vi "TI sbRIO Main (FPGA) (CMFB first try).vi"() -> ()   [LabVIEW 2019]
uses:
  <userlib>/_NI SPI IP/FPGA/Controllers/Public/Transfer Settings.ctl
  Type Defs/Diagnostic Mode.ctl
  Controls/SPI Channels.ctl
  <vilib>/Platform/TimedLoop/XDataNode/timing_clust.ctl
  <vilib>/Platform/TimedLoop/XDataNode/nitl_modes.ctl
  <vilib>/Platform/TimedLoop/XDataNode/wakeup.ctl
  <vilib>/rvi/FXPMathLib/FxpDiv/subVIs/nifxpmath_Div_SimConfig.ctl
  <vilib>/rvi/FXPMathLib/basic elements/FxpIntAccumulator/subVIs/nifxpmath_IntAccumulator_SimConfig.ctl
  <vilib>/rvi/FXPMathLib/FxpSqrt/subVIs/nifxpmath_Sqrt_SimConfig.ctl
  <vilib>/fxp/LVFixedPointOverflowPolicyTypeDef.ctl
  <userlib>/_NI SPI IP/FPGA/Controllers/Public/Spi Master Inputs.ctl
  <vilib>/rvi/Emulation/niFpgaGetClockAttributes.vi
  <vilib>/rvi/Emulation/niFpgaSctlEmulationGetInTimedLoop.vi
  <vilib>/rvi/Emulation/niFpgaEmulationReportErrorSimple.vi
  <vilib>/rvi/eio/common/nirviEmuTemplateMethod_errors.vi
  Onboard AIs Global.vi
  <vilib>/rvi/Emulation/niFpgaProcessEmulError.vi
  <vilib>/rvi/Emulation/niFpgaCriticalErrorInLSC.vi
  ADC AI Global.vi
  <vilib>/rvi/FXPMathLib/FxpDiv/simVIs/DllFxpDivTemp_sub.vi
  <vilib>/rvi/DataTransferAndStorage/Container/Common/niFpgaContainerExecOnDevCompGetState.vi
  <vilib>/rvi/Emulation/niFpgaEmulationIsFPGAContextNoSignature.vi
  <vilib>/rvi/errors/niFpgaSetErrorForExecOnDevCompSimple.vi
  <vilib>/rvi/eio/common/nirviEmuReportErrorAndStop.vi
  <vilib>/rvi/DataTransferAndStorage/Container/Common/niFpgaContainerGetUniqueNameForEmu.vi
  <vilib>/rvi/FIFO/Fifo_Resource/nirvififoEmulationSetSize.vi
  <vilib>/rvi/FIFO/Fifo_Resource/nirviFifoEmulationQueueMgr.vi
  <instcachedir>/0/nirviFifoEmulationQueueMgr_E5CAEC123FF24DC58D834DCA3CDAA9B5.lvgen/nirviFifoEmulationQueueMgr_E5CAEC123FF24DC58D834DCA3CDAA9B5_000.vi
  <vilib>/rvi/FIFO/Fifo_Resource/nirvififoEmulationDetermineInputValidOut.vi
  <vilib>/rvi/FIFO/Fifo_Resource/nirvififoEmulationCreateLock.vi
  <vilib>/rvi/FIFO/Fifo_Resource/nirvififoEmulationObtainLock.vi
  <vilib>/rvi/FIFO/Fifo_Resource/nirvififoEmulationReleaseLock.vi
  <vilib>/rvi/occurrence/nirviWaitOnOccurrenceBase.vi
  <vilib>/rvi/errors/nirviReportUnexpectedCaseInternalError.vi
  <vilib>/rvi/errors/nirviReportUnexpectedCaseInternalError (U32).vi
  <vilib>/Utility/error.llb/Clear Errors.vi
  <vilib>/rvi/interface/RandomDataEmulation/niFpgaRandomDataHandleErrors.vi
  Flow Frequencies Global.vi
  ADC AI Global (Avg).vi
  <vilib>/rvi/Analysis/common/codeGenErrors/XNode/niFpgaXNodeCodeGenErrorHandle.vi
  <vilib>/rvi/FXPMathLib/basic elements/FxpIntAccumulator/simVIs/DllFxpIntAccumulator_sub.vi
  <vilib>/rvi/FXPMathLib/FxpSqrt/simVIs/DllSqrtTemp_sub.vi
  Pump Currents Global.vi
  Diagnostic Global.vi
  <vilib>/eio/EIONode/EIONode.xnode
  <vilib>/rvi/FXPMathLib/FxpDiv/XNode/nifxpmath_Div.xnode
  <vilib>/rvi/DataTransferAndStorage/Container/XNode/niFpgaContainer.xnode
  <vilib>/rvi/FIFO/Fifo_Resource/niFpgaFifoEmulationRefIn.vi
  <vilib>/rvi/FXPMathLib/FxpMul/XNode/nifxpmath_Multiplier.xnode
  <vilib>/rvi/FXPMathLib/FxpAdd/XNode/nifxpmath_Add.xnode
  <vilib>/rvi/Analysis/measure/butterworth/XNode/niFpgaButterworthFilter.xnode
  <vilib>/rvi/Analysis/measure/dc-rms/XNode/niFpgaDC-RMS.xnode
  <vilib>/Platform/TimedLoop/XDataNode/XDataNode.xnode
  <vilib>/rvi/FXPMathLib/basic elements/FxpIntAccumulator/XNode/nifxpmath_IntAccumulator.xnode
  <vilib>/rvi/FXPMathLib/FxpSqrt/XNode/nifxpmath_Sqrt.xnode
  <vilib>/rvi/interface/RandomDataEmulation/nirviRandomDataFpgaReadWriteTemplate.vi
  <vilib>/eio/EIOMethodNode/EIOMethodNode.xnode
  <vilib>/rvi/FXPMathLib/sim/FxpSim.dll
  <vilib>/Platform/TimedLoop/XDataNode/XDNodeRunTimeDep.lvlib
  <userlib>/_NI SPI IP/FPGA/Controllers/NI SPI IP FPGA.lvlib
panel:
  out "Restarts":i32[](array[numeric])
  out "Cmd Pump Starts":u32[](array[numeric])
  in  "Stop Command":i32
  in  "Initial Cmd Starts":u32[](array[numeric])=[0, 0, 0, 0, 0, 0]
  in  "Ctrl Currents":fxp<+/-,28,17>[](array[numeric])=[0.0, 0.0, 0.0, 0.0, 0.0, 0.0]
  in  "Initial Acutal Starts":u32[](array[numeric])=[0, 0, 0, 0, 0, 0]
  in  "Power Relays":bool[](array[boolean])=[FALSE, FALSE, FALSE, FALSE, FALSE, FALSE]
  out "Actual Pump Starts":u32[](array[numeric])
  out "Timers (ms)":u32[](array[numeric])
  out "Pump On States":bool[](array[boolean])
  in  "Off Current Thresh":fxp<+/-,28,17>
  in  "Min Off Time":u32
  in  "On Current Thresh":fxp<+/-,28,17>
  in  "Min On Time":u32
  in  "Reset Pump Starts":bool
  in  "Pump Starts Enable":bool
  in  "Diag Max Period (ticks)":u32
  in  "Diagnostic Mode":T1=enum."PSA"
  in  "Duty (Ticks)":i32[](array[numeric])=[0, 0, 0, 0, 0, 0]
  out "Elapsed Times OUT":fxp<+,40,40>[](array[numeric])
  out "Data OUT":fxp<+/-,28,17>[](array[numeric])
  in  "Diagnostic Filter":u16=5
  in  "Invert Diagnostic":bool
  in  "Diagnostic Freq Coeff":i32
  in  "Count Off-Time":bool
  in  "Elapsed Times":fxp<+,40,40>[](array[numeric])=[0.0, 0.0, 0.0, 0.0, 0.0, 0.0]
  in  "ADC Init":bool=TRUE
  in  "FFT_Amp?":bool=TRUE
  in  "Max Period (ticks)":u32
  in  "Freq Flow?":bool
  in  "Divide Value":u8=1
  in  "Current Threshold":fxp<+,26,7>=1.0 format="%#_22g"
  in  "Enable Timers":bool[](array[boolean])=[FALSE, FALSE, FALSE, FALSE, FALSE, FALSE]
  in  "PumpCurrentM":fxp<+/-,16,9>=-60.0 format="%#_25g"
  in  "PumpCurrentB":fxp<+/-,16,9>=-60.0 format="%#_25g"
  in  "InvertPWM?":bool
  in  "DIO25":bool
  in  "DIO24":bool
  out "DIO23":bool
  in  "DIO22":bool
  in  "DIO21":bool
  in  "DIO20":bool
  in  "DIO19":bool
  in  "DIO18":bool
  in  "DIO17":bool
  in  "DIO16":bool
  in  "DIO15":bool
  in  "DIO14":bool
  in  "DIO13":bool
  in  "DIO12":bool
  out "ADC Read Data":u64 format="%.0x"
  in  "ADC CS Mode":enum16{"All", "CS0", "CS1"}(ring)
  in  "ADC Trigger":bool=TRUE
  in  "ADC SPI Settings":T2 {"Direction Change Bit" max=64 step=1; "Transfer Length (bits)" min=1 max=64 step=1}
  in  "ADC Data In":u64 format="%.0x"
  in  "ADC Conversion Request":bool
  in  "ADC Manual":bool
  in  "Brushless":bool
  in  "AI Divisor":u32
  in  "AO3":fxp<+/-,20,5>
  in  "AO2":fxp<+/-,20,5>
  in  "Pressure Cmd":fxp<+/-,20,5>
  in  "PS Cmd":fxp<+/-,20,5>
  in  "Loop Timer (uSec)":u32=100
  in  "Timer Resets":bool[](array[boolean])=[FALSE, FALSE, FALSE, FALSE, FALSE, FALSE]
  in  "PWM Period (Ticks)":u32=40000000
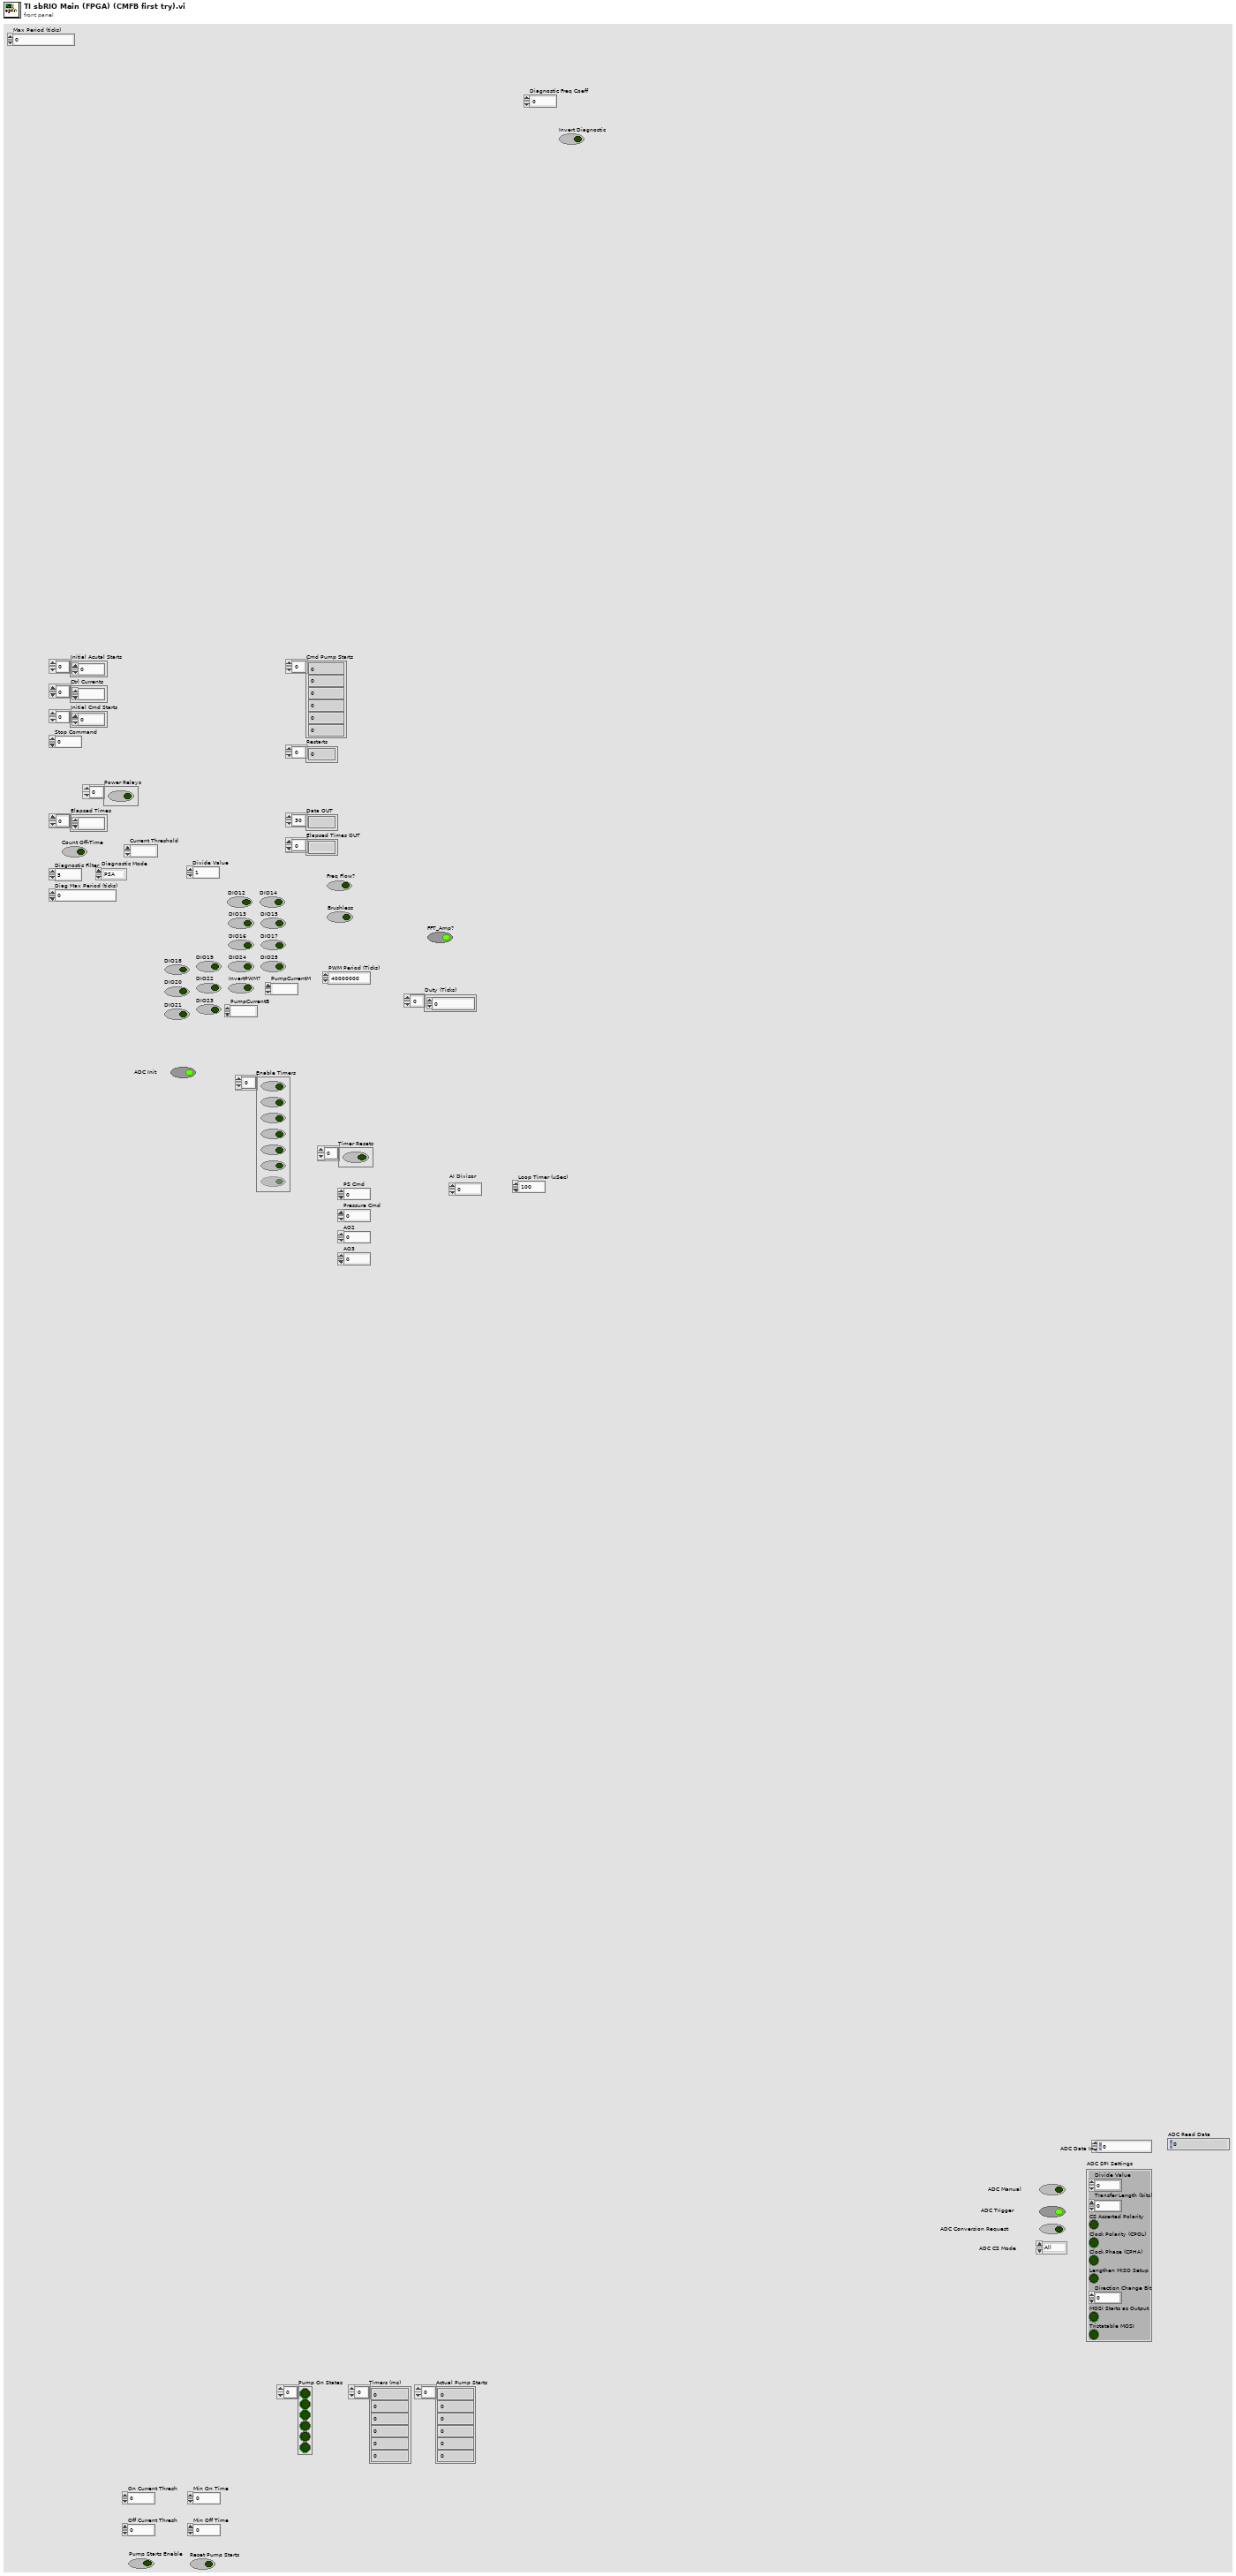
[diagram p1: front panel]
types:
  T1 = typedef "Diagnostic Mode.ctl" = enum16{"None", "PSA", "CMFB"}
  T2 = typedef "NI SPI IP FPGA.lvlib/Transfer Settings.ctl" = cluster{"Divide Value":u8, "Transfer Length (bits)":u8, "CS Asserted Polarity":bool, "Clock Polarity (CPOL)":bool, "Clock Phase (CPHA)":bool, "Lengthen MISO Setup":bool, "Direction Change Bit":u8, "MOSI Starts as Output":bool, "Tristatable MOSI":bool}
  T3 = typedef "SPI Channels.ctl" = cluster{"CS":refnum<k21>, "CLK":refnum<k21>, "MOSI":refnum<k21>, "MISO":refnum<k21>}
  T4 = typedef "XDNodeRunTimeDep.lvlib/timing_clust.ctl" = cluster{"Expected End [f-1]":u64, "Actual End [f-1]":u64, "Finished Late? [f-1]":bool, "Expected End [i-1]":u64, "Actual End [i-1]":u64, "Finished Late? [i-1]":bool, "Expected Start [i]":u64, "Actual Start [i]":u64, "Expected Start [f]":u64, "Actual Start [f]":u64, "Source Name":string, "Structure Name":string, "Period":i64, "Deadline":i64, "Offset":i64, "Start":i64, "Priority":i32, "Timeout":i32, "Mode":T5, "Wakeup Reason":T6, "Error":errorcluster, "Source Type":string, "Secondary Source Type":string, "Global End Time":u64, "Global Start Time":u64, "Frame Duration":u64, "Iteration Duration":u64, "Assigned CPU":i32, "I/O Scan Engine Mode":u32}
  T5 = typedef "XDNodeRunTimeDep.lvlib/nitl_modes.ctl" = enum32{"No Change", "Process missed periods, maintain original phase", "Discard missed periods, maintain original phase", "Process missed periods, ignore original phase", "Discard missed periods, ignore original phase"}
  T6 = typedef "XDNodeRunTimeDep.lvlib/wakeup.ctl" = enum32{"Normal", "Aborted", "Asynchronous wakeup", "Timing source error", "Timed loop error", "Timeout"}
  T7 = typedef "NI SPI IP FPGA.lvlib/Spi Master Inputs.ctl" = cluster{"MISO":bool}
  T8 = typedef "NI SPI IP FPGA.lvlib/Spi Master Outputs.ctl" = cluster{"Chip Select":bool, "Clock":bool, "MOSI":bool, "MOSI OE":bool}
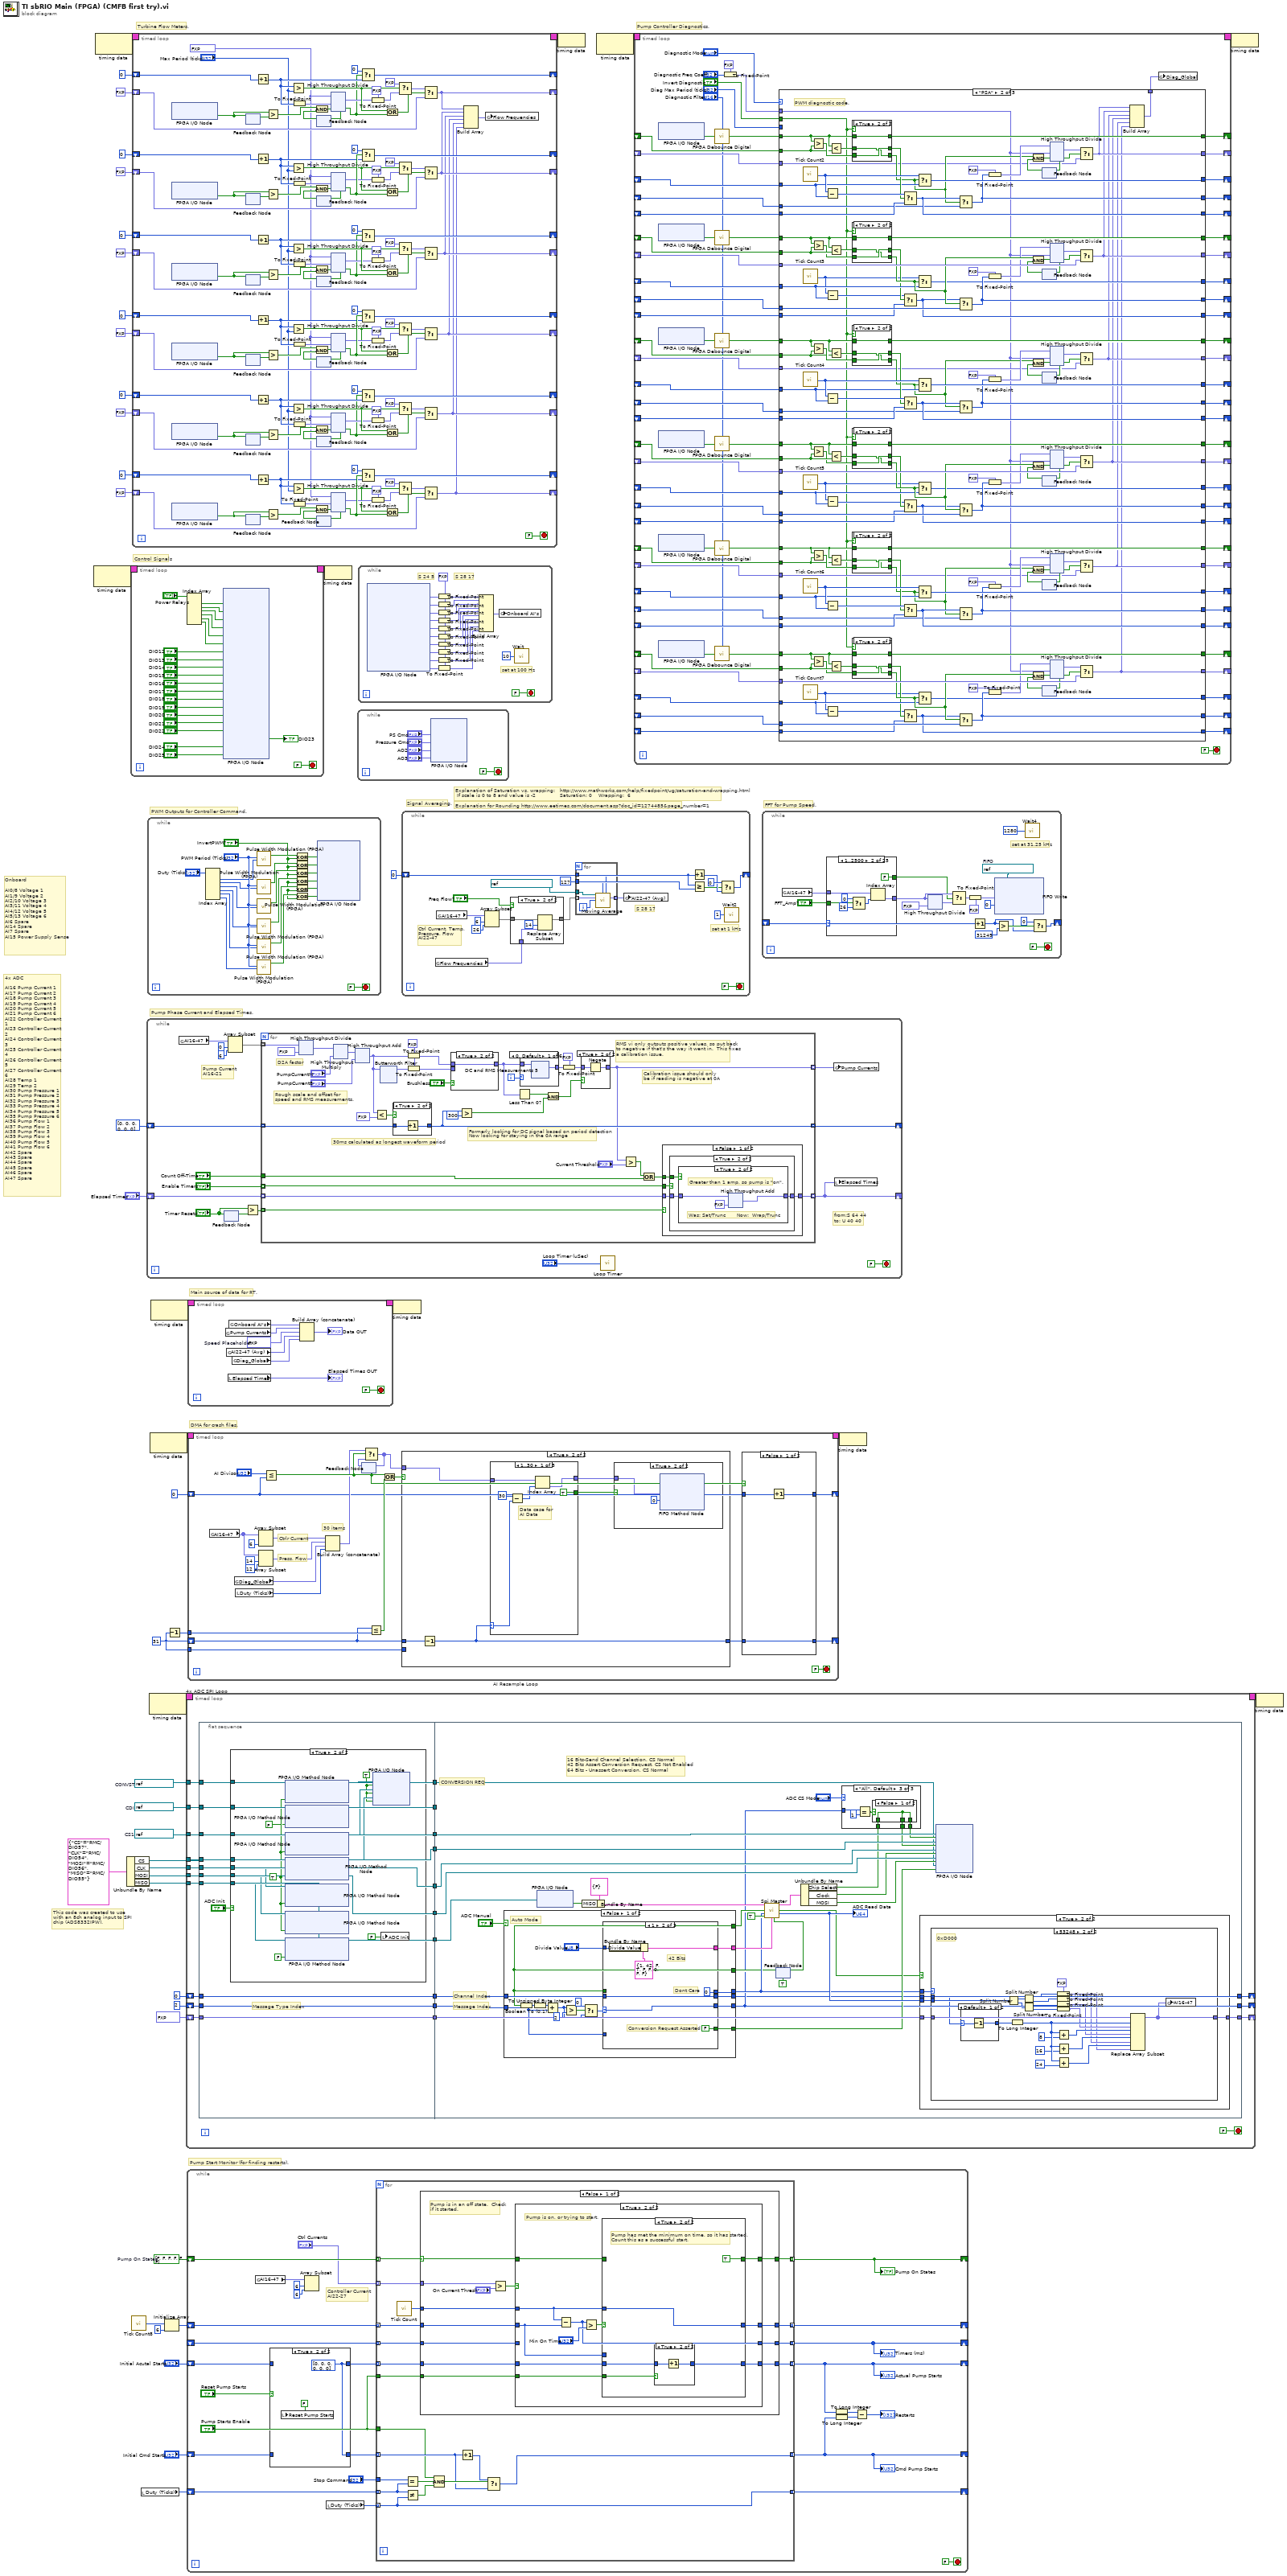
[diagram p0: block diagram]
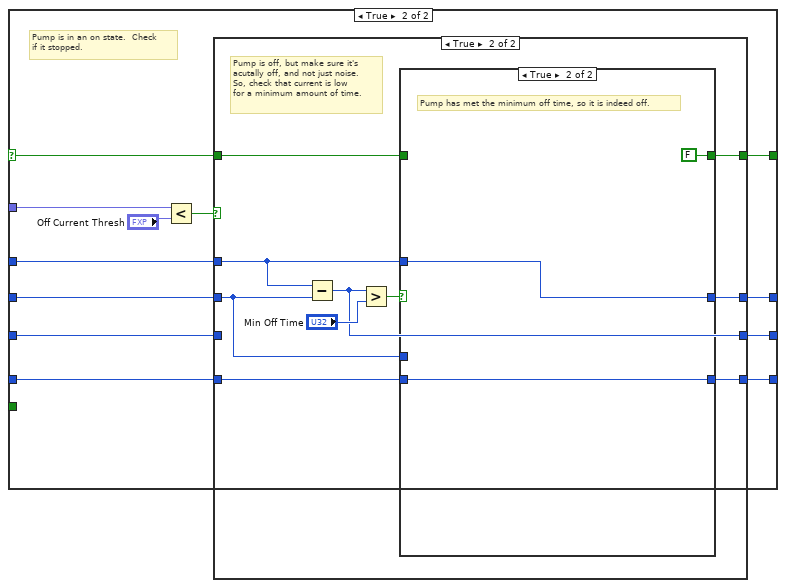
[diagram p6: hidden frame]
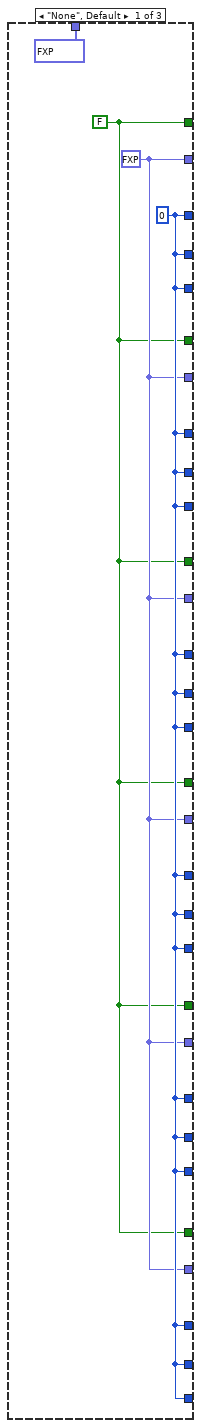
[diagram p9: hidden frame]
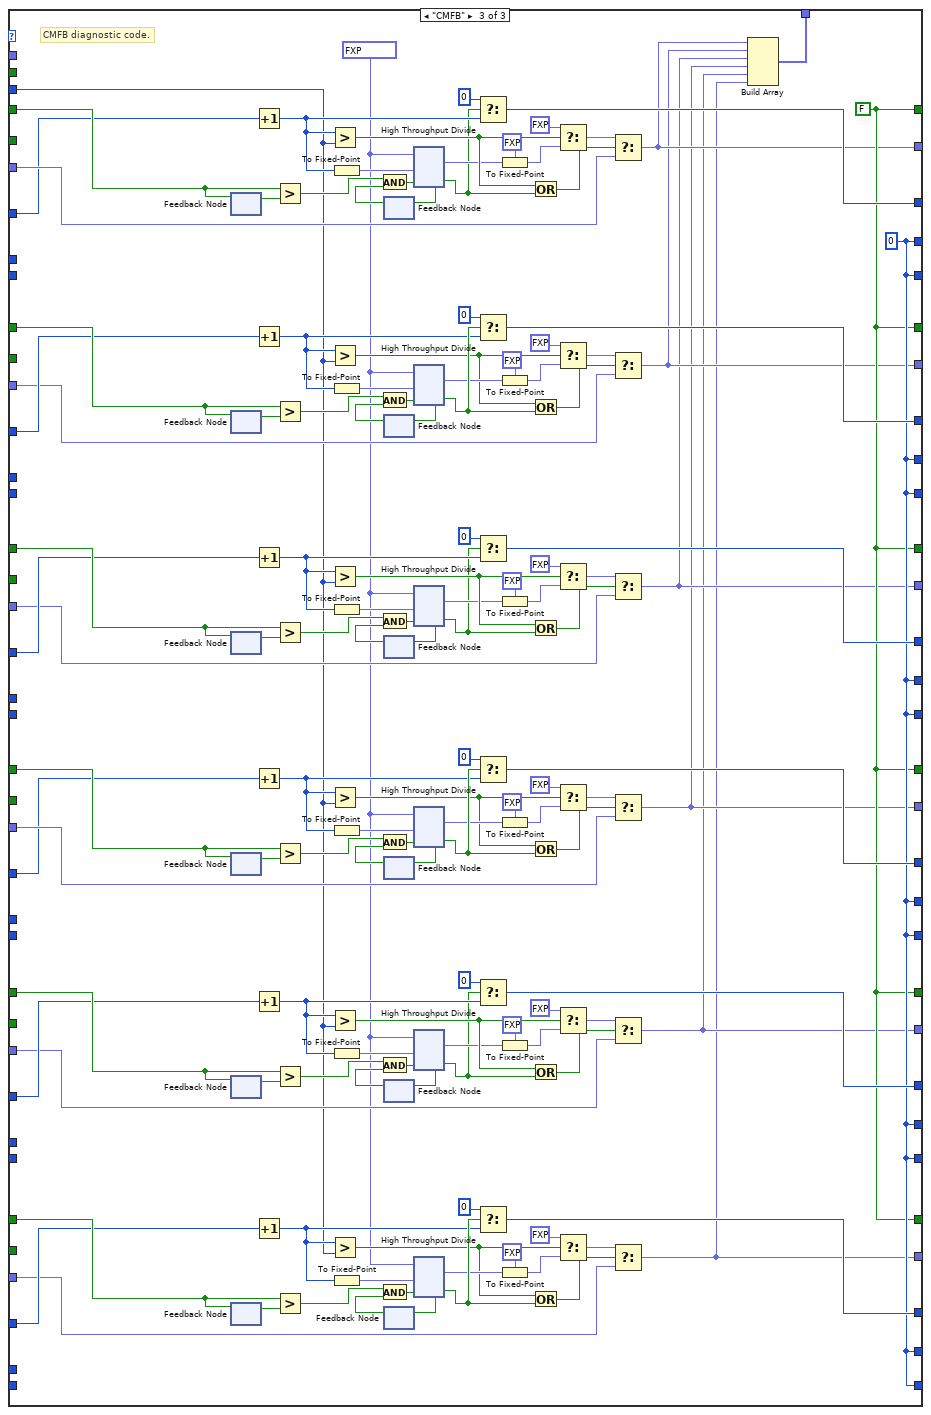
[diagram p16: hidden frame]
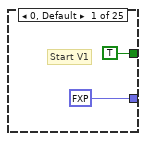
[diagram p17: hidden frame]
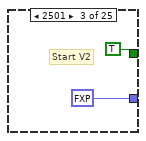
[diagram p18: hidden frame]
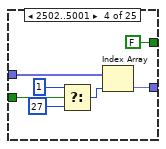
[diagram p19: hidden frame]
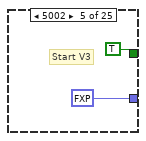
[diagram p20: hidden frame]
diagram:
  w7 = bool[] [FALSE, FALSE, FALSE, FALSE, FALSE, FALSE]  # Pump On States
  w38 = refnum<k21> "RMC/DIO60"  # CONVST
  w39 = refnum<k21> "RMC/DIO59"  # CDI
  w40 = refnum<k21> "RMC/DIO58"  # CS1
  w44 = u8 31 ("Sample Divisor")
  # "Pump Start Monitor (for finding restarts)."
  # "DMA for crash files."
  # "Main source of data for RT."
  # "Pump Phase Current and Elapsed Times."
  # "PWM Outputs for Controller Command."
  # "Signal Averaging."
  # "FFT for Pump Speed."
  # "Pump Controller Diagnostics."
  # "Turbine Flow Meters."
  # "Control Signals"
  # "4x ADC\n\nAI16\tPump Current 1\nAI17\tPump Current 2\nAI18\tPump Current 3\nAI19\tPump Current 4\nAI20\tPump Current 5\nAI21\tPump Current 6\nAI22\tController Current 1\nAI23\tController Current 2\nAI24\tController Current 3\nAI25\tController Current 4\nAI26\tController Current 5\nAI27\tController Current 6\nAI28\tTemp 1\nAI29\tTemp 2\nAI30\tPump Pressure 1\nAI31\tPump Pressure 2\nAI32\tPump Pressure 3\nAI33\tPump Pressure 4\nAI34\tPump Pressure 5\nAI35\tPump Pressure 6\nAI36\tPump Flow 1\nAI37\tPump Flow 2\nAI38\tPump Flow 3\nAI39\tPump Flow 4\nAI40\tPump Flow 5\nAI41\tPump Flow 6\nAI42\tSpare\nAI43\tSpare\nAI44\tSpare\nAI45\tSpare\nAI46\tSpare\nAI47\tSpare"
  # "Onboard\n\nAI0/8\tVoltage 1\nAI1/9\tVoltage 2\nAI2/10\tVoltage 3\nAI3/11\tVoltage 4\nAI4/12\tVoltage 5\nAI5/13\tVoltage 6\nAI6\tSpare\nAI14\tSpare\nAI7\tSpare\nAI15\tPower Supply Sense"
  # "This code was created to use\nwith an 8ch analog input to SPI\nchip (ADS8332IPW)."
  # "Explanation for Rounding http://www.eetimes.com/document.asp?doc_id=1274485&page_number=1"
  # "Explanation of Saturation vs. wrapping:   http://www.mathworks.com/help/fixedpoint/ug/saturation-and-wrapping.html\n If scale is 0 to 8 and value is -2               Saturation: 0    Wrapping:  6"
  n1 = node-c288() -> (w29:T4)  [unwired: 1 in]
  n2 = node-c288() -> (w27:T4)  [unwired: 1 in]
  n3 = Unbundle By Name(T3 {"CS"="RMC/DIO57", "CLK"="RMC/DIO54", "MOSI"="RMC/DIO56", "MISO"="RMC/DIO55"} ("SPI Channels")) -> ("CS"=w31:refnum<k21>, "CLK"=w32:refnum<k21>, "MOSI"=w33:refnum<k21>, "MISO"=w34:refnum<k21>)
  n4 = timed-loop {
    timing: w29 -> [_]
    timing-out: [_] -> w28
    stop <- FALSE stop-if-true
    n5 = Index Array(array="Power Relays") -> (element #1=w54:bool, element #2=w53:bool, element #3=w52:bool, element #4=w51:bool, element #5=w50:bool, element #6=w49:bool)  [unwired: 6 in]
    n6 = xnode "FPGA I/O Node"("RMC/DIO6"=w54, "RMC/DIO7"=w53, "RMC/DIO8"=w52, "RMC/DIO9"=w51, "RMC/DIO10"=w50, "RMC/DIO11"=w49, "RMC/DIO12"="DIO12", "RMC/DIO13"="DIO13", "RMC/DIO14"="DIO14", "RMC/DIO15"="DIO15", "RMC/DIO16"="DIO16", "RMC/DIO17"="DIO17", "RMC/DIO18"="DIO18", "RMC/DIO19"="DIO19", "RMC/DIO20"="DIO20", "RMC/DIO21"="DIO21", "RMC/DIO22"="DIO22", "RMC/DIO24"="DIO24", "RMC/DIO25"="DIO25") -> ("RMC/DIO23"=→"DIO23":bool)  [unwired: 21 in, 21 out]
  }
  n7 = call "Tick Count8"() -> ("Tick Count(mSec)"=w3:u32)
  n8 = timed-loop {
    timing: w27 -> [_]
    timing-out: [_] -> w26
    shift-right: [w197] -> _
    shift-left: u32 0 ("f") -> [w196]
    shift-right: [w79] -> _
    shift-left: fxp<+/-,28,17> 0.0 ("AI0") -> [w191]
    shift-right: [w166] -> _
    shift-left: u32 0 ("f") -> [w167]
    shift-right: [w78] -> _
    shift-left: fxp<+/-,28,17> 0.0 ("AI0") -> [w172]
    shift-right: [w157] -> _
    shift-left: u32 0 ("f") -> [w156]
    shift-right: [w77] -> _
    shift-left: fxp<+/-,28,17> 0.0 ("AI0") -> [w151]
    shift-right: [w126] -> _
    shift-left: u32 0 ("f") -> [w127]
    shift-right: [w76] -> _
    shift-left: fxp<+/-,28,17> 0.0 ("AI0") -> [w132]
    shift-right: [w117] -> _
    shift-left: u32 0 ("f") -> [w116]
    shift-right: [w75] -> _
    shift-left: fxp<+/-,28,17> 0.0 ("AI0") -> [w111]
    shift-right: [w86] -> _
    shift-left: u32 0 ("f") -> [w87]
    shift-right: [w74] -> _
    shift-left: fxp<+/-,28,17> 0.0 ("AI0") -> [w92]
    stop <- FALSE stop-if-true
    w81 = fxp<+,32,32> 40000000.0 ("x")
    n9 = xnode "FPGA I/O Node"() -> ("RMC/DIO32"=w201:bool)  [unwired: 1 in, 1 out]
    n10 = xnode "FPGA I/O Node"() -> ("RMC/DIO33"=w162:bool)  [unwired: 1 in, 1 out]
    n11 = xnode "FPGA I/O Node"() -> ("RMC/DIO34"=w161:bool)  [unwired: 1 in, 1 out]
    n12 = xnode "FPGA I/O Node"() -> ("RMC/DIO35"=w122:bool)  [unwired: 1 in, 1 out]
    n13 = xnode "FPGA I/O Node"() -> ("RMC/DIO36"=w121:bool)  [unwired: 1 in, 1 out]
    n14 = xnode "FPGA I/O Node"() -> ("RMC/DIO37"=w82:bool)  [unwired: 1 in, 1 out]
    n15 = feedback-in #1(w201) -> ()
    n16 = feedback #1() -> (w200:bool)  [unwired: 1 in]
    n17 = feedback #2() -> (w163:bool)  [unwired: 1 in]
    n18 = feedback-in #2(w162) -> ()
    n19 = feedback #3() -> (w160:bool)  [unwired: 1 in]
    n20 = feedback-in #3(w161) -> ()
    n21 = feedback #4() -> (w123:bool)  [unwired: 1 in]
    n22 = feedback-in #4(w122) -> ()
    n23 = feedback #5() -> (w120:bool)  [unwired: 1 in]
    n24 = feedback-in #5(w121) -> ()
    n25 = feedback #6() -> (w83:bool)  [unwired: 1 in]
    n26 = feedback-in #6(w82) -> ()
    n27 = Increment(x=w196) -> (x+1=w195:u32)
    n28 = Increment(x=w167) -> (x+1=w168:u32)
    n29 = Increment(x=w156) -> (x+1=w155:u32)
    n30 = Increment(x=w127) -> (x+1=w128:u32)
    n31 = Increment(x=w116) -> (x+1=w115:u32)
    n32 = Increment(x=w87) -> (x+1=w88:u32)
    n33 = Greater?(x=w201, y=w200) -> (0:w182:bool)
    n34 = Greater?(x=w162, y=w163) -> (0:w181:bool)
    n35 = Greater?(x=w161, y=w160) -> (0:w142:bool)
    n36 = Greater?(x=w122, y=w123) -> (0:w141:bool)
    n37 = Greater?(x=w121, y=w120) -> (0:w102:bool)
    n38 = Greater?(x=w82, y=w83) -> (0:w101:bool)
    n39 = Greater?(x=w195, y="Max Period (ticks)") -> (0:w199:bool)
    n40 = Greater?(x=w168, y="Max Period (ticks)") -> (0:w164:bool)
    n41 = Greater?(x=w155, y="Max Period (ticks)") -> (0:w159:bool)
    n42 = Greater?(x=w128, y="Max Period (ticks)") -> (0:w124:bool)
    n43 = Greater?(x=w115, y="Max Period (ticks)") -> (0:w119:bool)
    n44 = Greater?(x=w88, y="Max Period (ticks)") -> (0:w84:bool)
    n45 = To Fixed-Point(number=w195) -> (fixed-point=w194:fxp<+,32,32>)  [unwired: 1 in]
    n46 = To Fixed-Point(number=w168) -> (fixed-point=w169:fxp<+,32,32>)  [unwired: 1 in]
    n47 = To Fixed-Point(number=w155) -> (fixed-point=w154:fxp<+,32,32>)  [unwired: 1 in]
    n48 = To Fixed-Point(number=w128) -> (fixed-point=w129:fxp<+,32,32>)  [unwired: 1 in]
    n49 = To Fixed-Point(number=w115) -> (fixed-point=w114:fxp<+,32,32>)  [unwired: 1 in]
    n50 = To Fixed-Point(number=w88) -> (fixed-point=w89:fxp<+,32,32>)  [unwired: 1 in]
    n51 = feedback #7() -> (w183:bool)  [unwired: 1 in]
    n52 = And(x=w182, y=w183) -> (x .and. y?=w184:bool)
    n53 = feedback #8() -> (w180:bool)  [unwired: 1 in]
    n54 = And(x=w181, y=w180) -> (x .and. y?=w179:bool)
    n55 = feedback #9() -> (w143:bool)  [unwired: 1 in]
    n56 = And(x=w142, y=w143) -> (x .and. y?=w144:bool)
    n57 = feedback #10() -> (w140:bool)  [unwired: 1 in]
    n58 = And(x=w141, y=w140) -> (x .and. y?=w139:bool)
    n59 = feedback #11() -> (w103:bool)  [unwired: 1 in]
    n60 = And(x=w102, y=w103) -> (x .and. y?=w104:bool)
    n61 = feedback #12() -> (w100:bool)  [unwired: 1 in]
    n62 = And(x=w101, y=w100) -> (x .and. y?=w99:bool)
    n63 = xnode "High Throughput Divide"("x"=w81, "y"=w194, "input valid"=w184) -> ("x/y"=w190:fxp<+,28,17>, "output valid"=w186:bool, "ready for input"=w185:bool)  [unwired: 1 in]
    n64 = feedback-in #7(w185) -> ()
    n65 = xnode "High Throughput Divide"("x"=w81, "y"=w169, "input valid"=w179) -> ("x/y"=w173:fxp<+,28,17>, "output valid"=w177:bool, "ready for input"=w178:bool)  [unwired: 1 in]
    n66 = feedback-in #8(w178) -> ()
    n67 = xnode "High Throughput Divide"("x"=w81, "y"=w154, "input valid"=w144) -> ("x/y"=w150:fxp<+,28,17>, "output valid"=w146:bool, "ready for input"=w145:bool)  [unwired: 1 in]
    n68 = feedback-in #9(w145) -> ()
    n69 = xnode "High Throughput Divide"("x"=w81, "y"=w129, "input valid"=w139) -> ("x/y"=w133:fxp<+,28,17>, "output valid"=w137:bool, "ready for input"=w138:bool)  [unwired: 1 in]
    n70 = feedback-in #10(w138) -> ()
    n71 = xnode "High Throughput Divide"("x"=w81, "y"=w114, "input valid"=w104) -> ("x/y"=w110:fxp<+,28,17>, "output valid"=w106:bool, "ready for input"=w105:bool)  [unwired: 1 in]
    n72 = feedback-in #11(w105) -> ()
    n73 = xnode "High Throughput Divide"("x"=w81, "y"=w89, "input valid"=w99) -> ("x/y"=w93:fxp<+,28,17>, "output valid"=w97:bool, "ready for input"=w98:bool)  [unwired: 1 in]
    n74 = feedback-in #12(w98) -> ()
    n75 = Select(t=u32 0 ("f"), s=w186, f=w195) -> (s? t:f=w197:u32)
    n76 = Select(t=u32 0 ("f"), s=w177, f=w168) -> (s? t:f=w166:u32)
    n77 = Select(t=u32 0 ("f"), s=w146, f=w155) -> (s? t:f=w157:u32)
    n78 = Select(t=u32 0 ("f"), s=w137, f=w128) -> (s? t:f=w126:u32)
    n79 = Select(t=u32 0 ("f"), s=w106, f=w115) -> (s? t:f=w117:u32)
    n80 = Select(t=u32 0 ("f"), s=w97, f=w88) -> (s? t:f=w86:u32)
    n81 = To Fixed-Point(fixed-point type=fxp<+/-,28,17> 0.0 ("AI0"), number=w190) -> (fixed-point=w188:fxp<+/-,28,17>)
    n82 = To Fixed-Point(fixed-point type=fxp<+/-,28,17> 0.0 ("AI0"), number=w173) -> (fixed-point=w175:fxp<+/-,28,17>)
    n83 = To Fixed-Point(fixed-point type=fxp<+/-,28,17> 0.0 ("AI0"), number=w150) -> (fixed-point=w148:fxp<+/-,28,17>)
    n84 = To Fixed-Point(fixed-point type=fxp<+/-,28,17> 0.0 ("AI0"), number=w133) -> (fixed-point=w135:fxp<+/-,28,17>)
    n85 = To Fixed-Point(fixed-point type=fxp<+/-,28,17> 0.0 ("AI0"), number=w110) -> (fixed-point=w108:fxp<+/-,28,17>)
    n86 = To Fixed-Point(fixed-point type=fxp<+/-,28,17> 0.0 ("AI0"), number=w93) -> (fixed-point=w95:fxp<+/-,28,17>)
    n87 = Or(x=w199, y=w186) -> (x .or. y?=w192:bool)
    n88 = Or(x=w164, y=w177) -> (x .or. y?=w171:bool)
    n89 = Or(x=w159, y=w146) -> (x .or. y?=w152:bool)
    n90 = Or(x=w124, y=w137) -> (x .or. y?=w131:bool)
    n91 = Or(x=w119, y=w106) -> (x .or. y?=w112:bool)
    n92 = Or(x=w84, y=w97) -> (x .or. y?=w91:bool)
    n93 = Select(t=fxp<+/-,28,17> 0.0 ("AI0"), s=w199, f=w188) -> (s? t:f=w193:fxp<+/-,28,17>)
    n94 = Select(t=fxp<+/-,28,17> 0.0 ("AI0"), s=w164, f=w175) -> (s? t:f=w170:fxp<+/-,28,17>)
    n95 = Select(t=fxp<+/-,28,17> 0.0 ("AI0"), s=w159, f=w148) -> (s? t:f=w153:fxp<+/-,28,17>)
    n96 = Select(t=fxp<+/-,28,17> 0.0 ("AI0"), s=w124, f=w135) -> (s? t:f=w130:fxp<+/-,28,17>)
    n97 = Select(t=fxp<+/-,28,17> 0.0 ("AI0"), s=w119, f=w108) -> (s? t:f=w113:fxp<+/-,28,17>)
    n98 = Select(t=fxp<+/-,28,17> 0.0 ("AI0"), s=w84, f=w95) -> (s? t:f=w90:fxp<+/-,28,17>)
    n99 = Select(t=w193, s=w192, f=w191) -> (s? t:f=w79:fxp<+/-,28,17>)
    n100 = Select(t=w170, s=w171, f=w172) -> (s? t:f=w78:fxp<+/-,28,17>)
    n101 = Select(t=w153, s=w152, f=w151) -> (s? t:f=w77:fxp<+/-,28,17>)
    n102 = Select(t=w130, s=w131, f=w132) -> (s? t:f=w76:fxp<+/-,28,17>)
    n103 = Select(t=w113, s=w112, f=w111) -> (s? t:f=w75:fxp<+/-,28,17>)
    n104 = Select(t=w90, s=w91, f=w92) -> (s? t:f=w74:fxp<+/-,28,17>)
    n105 = Build Array(w79, w78, w77, w76, w75, w74) -> (w73:fxp<+/-,28,17>[])
    n106 = global write "Flow Frequencies Global.vi" "Flow Frequencies"(w73) -> ()
  }
  n107 = local read "Duty (Ticks)"() -> (w1:i32[])
  n108 = while {
    shift-right: [w380] -> _
    shift-left: "Elapsed Times" -> [w391]
    shift-right: [w381] -> _
    shift-left: u32[] [0, 0, 0, 0, 0, 0] -> [w382]
    stop <- FALSE stop-if-true
    # "Pump Current\nAI16-21"
    # "from:S 64 44\nto: U 40 40"
    n109 = global read "ADC AI Global.vi" "AI16-47"() -> (w384:fxp<+/-,28,17>[])
    n110 = feedback #13() -> (w389:bool[])  [unwired: 1 in]
    n111 = feedback-in #13("Timer Resets") -> ()
    n112 = Array Subset(array=w384, index=0, length=6) -> (w386:fxp<+/-,28,17>[])
    n113 = Greater?(x="Timer Resets", y=w389) -> (0:w392:bool[])
    n114 = for {
      tunnel: w386 -> [w426] mode=indexing
      tunnel: w392 -> [w428] mode=indexing
      tunnel: [w398] -> w383 mode=indexing
      tunnel: w391 -> [w423] mode=indexing
      tunnel: [w422] -> w380 mode=indexing
      tunnel: "Enable Timers" -> [w417] mode=indexing
      tunnel: w382 -> [w405] mode=indexing
      tunnel: [w400] -> w381 mode=indexing
      tunnel: "Count Off-Time" -> [w396]
      i -> [w427]
      w421 = fxp<+/-,26,7> 0.0 ("out")
      # "Formerly looking for DC signal based on period detection\nNow looking for staying in the 0A range"
      # "Calibration issue should only\nbe if reading is negative at 0A"
      # "30ms calculated as longest waveform period"
      # "RMS vi only outputs positive values, so put back to negative if that's the way it went in.  This fixes a calibration issue."
      # "D2A factor"
      # "Rough scale and offset for\nspeed and RMS measurements."
      n115 = xnode "High Throughput Divide"("x"=w426, "y"=fxp<+,14,14> 13107.0 ("Current Scale")) -> ("x/y"=w420:fxp<+/-,28,17>)
      n116 = xnode ("High Throughput Multiply")("x"=w420, "y"="PumpCurrentM") -> ("x*y"=w419:fxp<+/-,29,10>)
      n117 = xnode ("High Throughput Add")("x"=w419, "y"="PumpCurrentB") -> ("x+y"=w408:fxp<+/-,30,11>)
      n118 = Less?(x=w408, y=fxp<+/-,30,11> 0.25) -> (x < y?=w406:bool)
      n119 = xnode "Butterworth Filter"("input data"=w408) -> ("output data"=w410:fxp<+/-,20,15>)  [unwired: 2 in, 1 out]
      n120 = case shown="True" w406 {
        tunnel: w405 -> [_ w431]
        tunnel: [u32 0 w430] -> w400
        frame False {
        }
        frame True {
          n121 = Increment(x=w431) -> (x+1=w430:u32)
        }
      }
      n122 = To Fixed-Point(fixed-point type=w421, number=w408) -> (fixed-point=w413:fxp<+/-,26,7>)
      n123 = To Fixed-Point(fixed-point type=w421, number=w410) -> (fixed-point=w411:fxp<+/-,26,7>)
      n124 = case shown="True" "Brushless" {
        tunnel: [w432 w433] -> w412
        tunnel: w413 -> [_ w433]
        tunnel: w411 -> [w432 _]
        frame False {
        }
        frame True {
        }
      }
      n125 = Greater?(x=w400, y=u32 300) -> (0:w401:bool)
      n126 = Less Than 0?(x=w412) -> (x < 0?=w404:bool)
      n127 = case shown="0, Default" w427 {
        tunnel: [w487 w597 w707 w817 w927 w1037] -> w414
        tunnel: w412 -> [w486 w596 w706 w816 w926 w1036]
        frame 0, Default {
          n128 = xnode ("DC and RMS Measurements 5")("input data"=w486) -> ("RMS"=w487:fxp<+,26,7>)  [unwired: 1 in, 1 out]
        }
        frame 1 {
          n129 = xnode ("DC and RMS Measurements")("input data"=w596) -> ("RMS"=w597:fxp<+,26,7>)  [unwired: 1 in, 1 out]
        }
        frame 2 {
          n130 = xnode ("DC and RMS Measurements 2")("input data"=w706) -> ("RMS"=w707:fxp<+,26,7>)  [unwired: 1 in, 1 out]
        }
        frame 3 {
          n131 = xnode ("DC and RMS Measurements 3")("input data"=w816) -> ("RMS"=w817:fxp<+,26,7>)  [unwired: 1 in, 1 out]
        }
        frame 4 {
          n132 = xnode ("DC and RMS Measurements 4")("input data"=w926) -> ("RMS"=w927:fxp<+,26,7>)  [unwired: 1 in, 1 out]
        }
        frame 5 {
          n133 = xnode ("DC and RMS Measurements 6")("input data"=w1036) -> ("RMS"=w1037:fxp<+,26,7>)  [unwired: 1 in, 1 out]
        }
      }
      n134 = And(x=w404, y=w401) -> (x .and. y?=w403:bool)
      n135 = To Fixed-Point(fixed-point type=fxp<+/-,28,17> 0.0 ("out"), number=w414) -> (fixed-point=w415:fxp<+/-,28,17>)
      n136 = case shown="True" w403 {
        tunnel: w415 -> [w434 w436]
        tunnel: [w434 w435] -> w398
        frame False {
        }
        frame True {
          n137 = Negate(x=w436) -> (-x=w435:fxp<+/-,29,18>)
        }
      }
      n138 = Greater?(x=w398, y="Current Threshold") -> (0:w397:bool)
      n139 = Or(x=w397, y=w396) -> (x .or. y?=w395:bool)
      n140 = case shown="False" w428 {
        tunnel: w395 -> [w467 _]
        tunnel: w423 -> [w466 _]
        tunnel: [w465 fxp<+,40,40> 0.0 ("AI0")] -> w422
        tunnel: w417 -> [w464 _]
        frame False {
          n141 = case shown="True" w464 {
            tunnel: w467 -> [_ w471]
            tunnel: w466 -> [w468 w470]
            tunnel: [w468 w469] -> w465
            frame False {
            }
            frame True {
              n142 = case shown="True" w471 {
                tunnel: [w472 w473] -> w469
                tunnel: w470 -> [w472 w475]
                frame False {
                }
                frame True {
                  # "Was: Sat/Trunc       Now:  Wrap/Trunc"
                  # "Greater than 1 amp, so pump is \"on\"."
                  n143 = xnode ("High Throughput Add")("x"=w475, "y"=fxp<+,1,1> 1.0) -> ("x+y"=w473:fxp<+,40,40>)
                }
              }
            }
          }
        }
        frame True {
        }
      }
    }
    n144 = call "Loop Timer"("Count(uSec)"="Loop Timer (uSec)") -> ()  [unwired: 1 out]
    n145 = global write "Pump Currents Global.vi" "Pump Currents"(w383) -> ()
    n146 = local write "Elapsed Times"(w380) -> ()
  }
  n147 = while {
    stop <- FALSE stop-if-true
    n148 = Index Array(array="Duty (Ticks)") -> (element #1=w1151:i32, element #2=w1150:i32, element #3=w1149:i32, element #4=w1148:i32, element #5=w1147:i32, element #6=w1146:i32)  [unwired: 6 in]
    n149 = call "Pulse Width Modulation (FPGA).vi"("PWM Period (Ticks)"="PWM Period (Ticks)", "PWM Duty Cycle (Ticks)"=w1151) -> ("PWM DO"=w1165:bool)  [unwired: 14 in, 3 out]
    n150 = call "Pulse Width Modulation (FPGA).vi"("PWM Period (Ticks)"="PWM Period (Ticks)", "PWM Duty Cycle (Ticks)"=w1150) -> ("PWM DO"=w1164:bool)  [unwired: 14 in, 3 out]
    n151 = call "Pulse Width Modulation (FPGA).vi"("PWM Period (Ticks)"="PWM Period (Ticks)", "PWM Duty Cycle (Ticks)"=w1149) -> ("PWM DO"=w1163:bool)  [unwired: 14 in, 3 out]
    n152 = call "Pulse Width Modulation (FPGA).vi"("PWM Period (Ticks)"="PWM Period (Ticks)", "PWM Duty Cycle (Ticks)"=w1148) -> ("PWM DO"=w1162:bool)  [unwired: 14 in, 3 out]
    n153 = call "Pulse Width Modulation (FPGA).vi"("PWM Period (Ticks)"="PWM Period (Ticks)", "PWM Duty Cycle (Ticks)"=w1147) -> ("PWM DO"=w1161:bool)  [unwired: 14 in, 3 out]
    n154 = call "Pulse Width Modulation (FPGA).vi"("PWM Period (Ticks)"="PWM Period (Ticks)", "PWM Duty Cycle (Ticks)"=w1146) -> ("PWM DO"=w1160:bool)  [unwired: 14 in, 3 out]
    n155 = Exclusive Or(1:"InvertPWM?", 2:w1165) -> (0:w1158:bool)
    n156 = Exclusive Or(1:"InvertPWM?", 2:w1164) -> (0:w1157:bool)
    n157 = Exclusive Or(1:"InvertPWM?", 2:w1163) -> (0:w1156:bool)
    n158 = Exclusive Or(1:"InvertPWM?", 2:w1162) -> (0:w1155:bool)
    n159 = Exclusive Or(1:"InvertPWM?", 2:w1161) -> (0:w1154:bool)
    n160 = Exclusive Or(1:"InvertPWM?", 2:w1160) -> (0:w1153:bool)
    n161 = xnode "FPGA I/O Node"("RMC/DIO0"=w1158, "RMC/DIO1"=w1157, "RMC/DIO2"=w1156, "RMC/DIO3"=w1155, "RMC/DIO4"=w1154, "RMC/DIO5"=w1153) -> ()  [unwired: 7 in, 7 out]
  }
  n162 = node-c288() -> (w42:T4)  [unwired: 1 in]
  n163 = node-c288() -> (w48:T4)  [unwired: 1 in]
  n164 = node-c288() -> (w9:T4)  [unwired: 1 in]
  n165 = Initialize Array(w3, 6 ("dimension size")) -> (w5:u32[])
  n166 = Decrement(x=w44) -> (x-1=w45:u8)
  n167 = timed-loop "4x ADC SPI Loop" {
    shift-right: [w1189] -> _
    shift-left: fxp<+/-,28,17>[] [0.0, 0.0, 0.0, 0.0, 0.0, 0.0, 0.0, 0.0, 0.0, 0.0, 0.0, 0.0, 0.0, 0.0, 0.0, 0.0, 0.0, 0.0, 0.0, 0.0, 0.0, 0.0, 0.0, 0.0, 0.0, 0.0, 0.0, 0.0, 0.0, 0.0, 0.0, 0.0] -> [w1190]
    tunnel: w31 -> [w1188]
    tunnel: w32 -> [w1187]
    tunnel: w33 -> [w1186]
    tunnel: w34 -> [w1185]
    tunnel: w40 -> [w1184]
    tunnel: w38 -> [w1183]
    tunnel: w39 -> [w1182]
    timing: w42 -> [_]
    timing-out: [_] -> w41
    shift-right: [w1171] -> _
    shift-left: u8 2 ("lo(x)") -> [w1172]
    shift-right: [w1168] -> _
    shift-left: u8 0 ("lo(x)") -> [w1169]
    stop <- FALSE stop-if-true
    n168 = flat-sequence {
      tunnel: [w1202] -> w1181
      tunnel: w1190 -> [w1202]
      tunnel: w1188 -> [w1201]
      tunnel: w1187 -> [w1200]
      tunnel: w1186 -> [w1199]
      tunnel: w1185 -> [w1198]
      tunnel: [w1201] -> w1180
      tunnel: [w1200] -> w1179
      tunnel: [w1199] -> w1178
      tunnel: [w1198] -> w1177
      tunnel: w1184 -> [w1197]
      tunnel: w1183 -> [w1196]
      tunnel: w1182 -> [w1195]
      tunnel: [w1197] -> w1176
      tunnel: [w1195] -> w1175
      tunnel: [w1196] -> w1174
      tunnel: [w1194] -> w1173
      tunnel: w1172 -> [w1194]
      tunnel: [w1193] -> w1170
      tunnel: w1169 -> [w1193]
      tunnel: w1181 -> [w1245]
      tunnel: [w1244] -> w1189
      tunnel: w1180 -> [w1240]
      tunnel: w1179 -> [w1243]
      tunnel: w1178 -> [w1242]
      tunnel: w1177 -> [w1241]
      tunnel: w1176 -> [w1239]
      tunnel: w1175 -> [_]
      tunnel: w1174 -> [w1225]
      tunnel: w1173 -> [w1226]
      tunnel: [w1220] -> w1171
      tunnel: w1170 -> [w1219]
      tunnel: [w1218] -> w1168
      frame #0 {
        # "Message Type Index"
        n169 = case shown="True" "ADC Init" {
          tunnel: w1201 -> [_ w1217]
          tunnel: w1200 -> [_ w1216]
          tunnel: w1199 -> [_ w1215]
          tunnel: w1198 -> [_ w1214]
          tunnel: w1197 -> [_ w1213]
          tunnel: w1196 -> [_ w1212]
          tunnel: w1195 -> [_ w1211]
          frame False {
          }
          frame True {
            w1204 = TRUE ("I/O Item")
            w1209 = TRUE ("Enable")
            n170 = xnode "FPGA I/O Method Node"("FPGA I/O In"=w1212, "Enable"=w1209) -> ("FPGA I/O Out"=w1205:refnum<k21>)
            n171 = xnode "FPGA I/O Method Node"("FPGA I/O In"=w1211, "Enable"=FALSE) -> ()  [unwired: 1 out]
            n172 = xnode "FPGA I/O Method Node"("FPGA I/O In"=w1213, "Enable"=w1209) -> ("FPGA I/O Out"=w1208:refnum<k21>)
            n173 = xnode "FPGA I/O Method Node"("FPGA I/O In"=w1217, "Enable"=w1209) -> ("FPGA I/O Out"=w1207:refnum<k21>)
            n174 = xnode "FPGA I/O Method Node"("FPGA I/O In"=w1216, "Enable"=w1209) -> ()  [unwired: 1 out]
            n175 = xnode "FPGA I/O Method Node"("FPGA I/O In"=w1215, "Enable"=w1209) -> ()  [unwired: 1 out]
            n176 = xnode "FPGA I/O Method Node"("FPGA I/O In"=w1214, "Enable"=FALSE) -> ()  [unwired: 1 out]
            n177 = xnode "FPGA I/O Node"("I/O Item"=w1204, "FPGA I/O In"=w1205, "I/O Item"=w1204, "FPGA I/O In"=w1208, "I/O Item"=w1204, "FPGA I/O In"=w1207) -> ()  [unwired: 3 out]
            n178 = local write "ADC Init"(FALSE ("ADC Init")) -> ()
          }
        }
      }
      frame #1 {
        # "Message Index"
        # "Channel Index"
        # "16 Bits-Send Channel Selection, CS Normal \n42 Bits Assert Conversion Request, CS Not Enabled\n64 Bits - Unassert Conversion, CS Normal"
        # "CONVERSION REQ"
        n179 = xnode "FPGA I/O Node"("FPGA I/O In"=w1241) -> ("I/O Item"=w1246:bool)  [unwired: 1 out]
        n180 = Bundle By Name(cluster=T7 {"MISO"=FALSE} ("spi input"), "MISO"=w1246) -> (w1247:T7)
        n181 = feedback #14(TRUE ("Chip Select")) -> (w1222:bool)
        n182 = case shown="False" "ADC Manual" {
          tunnel: w1222 -> [w1254 w1307]
          tunnel: [w1254 w1306] -> w1228
          tunnel: [w1259 "ADC SPI Settings"] -> w1227
          tunnel: w1226 -> [w1253 _]
          tunnel: [w1255 "ADC Data In"] -> w1223
          tunnel: [w1252 w1302] -> w1220
          tunnel: [w1258 "ADC Conversion Request"] -> w1224
          tunnel: w1219 -> [w1257 _]
          tunnel: [w1256 w1302] -> w1218
          frame False {
            # "Auto Mode"
            n183 = Boolean To (0,1)(Boolean=w1254) -> (0, 1=w1266:i16)
            n184 = To Unsigned Byte Integer(number=w1266) -> (unsigned 8bit integer=w1265:u8)
            n185 = Add(x=w1265, y=w1253) -> (x+y=w1261:u8)
            n186 = Greater?(x=w1261, y=u8 2) -> (0:w1263:bool)
            n187 = Select(t=u8 0 ("y"), s=w1263, f=w1261) -> (s? t:f=w1260:u8)
            n188 = case shown="1" w1260 {
              selector: w1260 -> [w1273 w1279 w1289]
              tunnel: [w1267 w1276 w1283] -> w1259
              tunnel: [TRUE ("I/O Item") FALSE ("I/O Item") TRUE ("I/O Item")] -> w1258
              tunnel: w1257 -> [w1272 w1280 w1288]
              tunnel: [w1272 w1280 w1287] -> w1256
              tunnel: [w1270 u64 0 u64 53248] -> w1255
              tunnel: w1254 -> [_ _ w1291]
              tunnel: w1253 -> [_ _ w1286]
              tunnel: [w1273 w1279 w1290] -> w1252
              tunnel: "Divide Value" -> [w1268 w1278 w1285]
              frame 0, Default {
                # "16 Bits"
                # "Channel Select"
                # "0x#000"
                n189 = Bundle By Name(cluster=T2 {"Divide Value"=1, "Transfer Length (bits)"=16, "CS Asserted Polarity"=FALSE, "Clock Polarity (CPOL)"=TRUE, "Clock Phase (CPHA)"=FALSE, "Lengthen MISO Setup"=FALSE, "Direction Change Bit"=0, "MOSI Starts as Output"=FALSE, "Tristatable MOSI"=FALSE} ("Master Settings 2"), "Divide Value"=w1268) -> (w1267:T2)
                n190 = To Unsigned Quad Integer(1:w1272) -> (0:w1271:u64)
                n191 = Logical Shift(y=i16 12, x=w1271) -> (x << y=w1270:u64)
              }
              frame 1 {
                # "Conversion Request Asserted"
                # "42 Bits"
                # "Dont Care"
                n192 = Bundle By Name(cluster=T2 {"Divide Value"=1, "Transfer Length (bits)"=42, "CS Asserted Polarity"=FALSE, "Clock Polarity (CPOL)"=TRUE, "Clock Phase (CPHA)"=FALSE, "Lengthen MISO Setup"=FALSE, "Direction Change Bit"=0, "MOSI Starts as Output"=FALSE, "Tristatable MOSI"=FALSE} ("Master Settings 2"), "Divide Value"=w1278) -> (w1276:T2)
              }
              frame 2 {
                # "64 Bits"
                # "Read CMD"
                n193 = Bundle By Name(cluster=T2 {"Divide Value"=1, "Transfer Length (bits)"=64, "CS Asserted Polarity"=FALSE, "Clock Polarity (CPOL)"=TRUE, "Clock Phase (CPHA)"=FALSE, "Lengthen MISO Setup"=FALSE, "Direction Change Bit"=0, "MOSI Starts as Output"=FALSE, "Tristatable MOSI"=FALSE} ("Master Settings 2"), "Divide Value"=w1285) -> (w1283:T2)
                n194 = case shown="False" w1291 {
                  tunnel: [w1294 w1298] -> w1290
                  tunnel: w1289 -> [_ w1298]
                  tunnel: w1288 -> [w1295 w1299]
                  tunnel: [w1295 w1296] -> w1287
                  tunnel: w1286 -> [w1294 _]
                  frame False {
                  }
                  frame True {
                    n195 = Increment(x=w1299) -> (x+1=w1297:u8)
                    n196 = case shown="8" w1297 {
                      selector: w1297 -> [w1300 _]
                      tunnel: [w1300 u8 0] -> w1296
                      frame Default {
                      }
                      frame 8 {
                      }
                    }
                  }
                }
              }
            }
          }
          frame True {
            w1302 = u8 0 ("y")
            # "Manual Mode"
            n197 = feedback #15(FALSE) -> (w1311:bool)
            n198 = feedback-in #15("ADC Trigger") -> ()
            n199 = Greater?(x="ADC Trigger", y=w1311) -> (0:w1308:bool)
            n200 = And(x=w1308, y=w1307) -> (x .and. y?=w1306:bool)
          }
        }
        n201 = call <userlib>:"Spi Master.vi"("spi input"=w1247, "start strobe"=w1228, "data to write"=w1223, "MOSI output enable done"=TRUE, "spi transfer settings"=w1227) -> ("spi output"=w1250:T8, "read data valid"=w1221:bool, "read data"=w1235:u64, "ready for input"=w1237:bool)  [unwired: 7 in]
        "ADC Read Data" <- w1235
        n202 = feedback-in #14(w1237) -> ()
        n203 = Unbundle By Name(w1250) -> ("Chip Select"=w1232:bool, "Clock"=w1236:bool, "MOSI"=w1249:bool)
        n204 = case shown="\"All\", Default" "ADC CS Mode" {
          tunnel: w1232 -> [w1313 w1315 w1319]
          tunnel: [TRUE ("Chip Select") w1315 w1318] -> w1231
          tunnel: [w1313 TRUE ("Chip Select") w1317] -> w1230
          tunnel: w1220 -> [_ _ w1321]
          frame "CS1" {
          }
          frame "CS0" {
          }
          frame "All", Default {
            n205 = Equal?(x=w1321, y=u8 1) -> (x = y?=w1316:bool)
            n206 = case shown="False" w1316 {
              tunnel: w1319 -> [w1322 _]
              tunnel: [w1322 w1323] -> w1318
              tunnel: [w1322 w1323] -> w1317
              frame False {
              }
              frame True {
                w1323 = TRUE ("Chip Select")
              }
            }
          }
        }
        n207 = case shown="True" w1221 {
          tunnel: w1235 -> [_ w1329]
          tunnel: w1245 -> [w1324 w1328]
          tunnel: [w1324 w1327] -> w1244
          tunnel: w1223 -> [_ w1326]
          tunnel: w1218 -> [_ w1325]
          frame False {
          }
          frame True {
            n208 = case shown="53248" w1326 {
              tunnel: w1329 -> [_ w1353]
              tunnel: w1328 -> [w1330 w1352]
              tunnel: [w1330 w1331] -> w1327
              tunnel: w1325 -> [_ w1341]
              frame Default {
              }
              frame 53248 {
                w1340 = fxp<+/-,28,17> 0.0 ("AI0")
                # "0xD000"
                n209 = case shown="Default" w1341 {
                  selector: w1341 -> [w1354 _]
                  tunnel: [w1355 u8 7] -> w1342
                  frame Default {
                    n210 = Decrement(x=w1354) -> (x-1=w1355:u8)
                  }
                  frame 0 {
                  }
                }
                n211 = Split Number(x=w1353) -> (hi(x)=w1351:u32, lo(x)=w1350:u32)
                n212 = To Long Integer(number=w1342) -> (32bit integer=w1349:i32)
                n213 = Split Number(x=w1351) -> (hi(x)=w1336:u16, lo(x)=w1337:u16)
                n214 = Split Number(x=w1350) -> (hi(x)=w1338:u16, lo(x)=w1339:u16)
                n215 = To Fixed-Point(fixed-point type=w1340, number=w1336) -> (fixed-point=w1332:fxp<+/-,28,17>)
                n216 = To Fixed-Point(fixed-point type=w1340, number=w1337) -> (fixed-point=w1333:fxp<+/-,28,17>)
                n217 = To Fixed-Point(fixed-point type=w1340, number=w1338) -> (fixed-point=w1334:fxp<+/-,28,17>)
                n218 = To Fixed-Point(fixed-point type=w1340, number=w1339) -> (fixed-point=w1335:fxp<+/-,28,17>)
                n219 = Add(x=w1349, y=8) -> (x+y=w1347:i32)
                n220 = Add(x=w1349, y=16) -> (x+y=w1346:i32)
                n221 = Add(x=w1349, y=24) -> (x+y=w1345:i32)
                n222 = Replace Array Subset(array=w1352, new element #1=w1335, index #1=w1349, new element #2=w1334, index #2=w1347, new element #3=w1333, index #3=w1346, new element #4=w1332, index #4=w1345) -> (w1331:fxp<+/-,28,17>[])
                n223 = global write "ADC AI Global.vi" "AI16-47"(w1331) -> ()
              }
            }
          }
        }
        n224 = xnode "FPGA I/O Node"("I/O Item"=w1230, "FPGA I/O In"=w1239, "I/O Item"=w1231, "FPGA I/O In"=w1240, "I/O Item"=w1236, "FPGA I/O In"=w1243, "I/O Item"=w1249, "FPGA I/O In"=w1242, "I/O Item"=w1224, "FPGA I/O In"=w1225) -> ()  [unwired: 5 out]
      }
    }
  }
  n225 = while {
    shift-right: [w1380] -> _
    shift-left: w5 -> [w1383]
    shift-right: [w1366] -> _
    shift-left: "Initial Acutal Starts" -> [w1377]
    shift-right: [w1381] -> _
    shift-left: w7 -> [w1382]
    shift-right: [w1379] -> _
    shift-left: _ -> [w1378]
    shift-right: [w1364] -> _
    shift-left: "Initial Cmd Starts" -> [w1359]
    shift-right: [w1367] -> _
    shift-left: w1 -> [w1370]
    stop <- FALSE stop-if-true
    # "Controller Current\nAI22-27"
    n226 = global read "ADC AI Global.vi" "AI16-47"() -> (w1372:fxp<+/-,28,17>[])
    n227 = case shown="True" "Reset Pump Starts" {
      tunnel: w1377 -> [w1386 _]
      tunnel: [w1386 w1388] -> w1375
      tunnel: [w1385 w1388] -> w1360
      tunnel: w1359 -> [w1385 _]
      frame False {
      }
      frame True {
        w1388 = u32[] [0, 0, 0, 0, 0, 0] ("Pump Starts")
        n228 = local write "Reset Pump Starts"(FALSE ("Reset Pump Starts")) -> ()
      }
    }
    n229 = Array Subset(array=w1372, index=6, length=6) -> ()  [unwired: 1 out]
    n230 = local read "Duty (Ticks)"() -> (w1369:i32[])
    n231 = for {
      tunnel: "Ctrl Currents" -> [w1409] mode=indexing
      tunnel: w1383 -> [w1408] mode=indexing
      tunnel: w1375 -> [w1407] mode=indexing
      tunnel: [w1406] -> w1366 mode=indexing
      tunnel: w1382 -> [w1404] mode=indexing
      tunnel: [w1405] -> w1381 mode=indexing
      tunnel: [w1402] -> w1380 mode=indexing
      tunnel: [w1401] -> w1379 mode=indexing
      tunnel: w1378 -> [w1400] mode=indexing
      tunnel: "Pump Starts Enable" -> [w1399]
      tunnel: w1360 -> [w1392] mode=indexing
      tunnel: w1370 -> [w1397] mode=indexing
      tunnel: w1369 -> [w1390] mode=indexing
      tunnel: "Stop Command" -> [w1398]
      tunnel: [w1391] -> w1364 mode=indexing
      tunnel: [w1390] -> w1367 mode=indexing
      tunnel: "Pump Starts Enable" -> [w1389]
      n232 = call "Tick Count"() -> ("Tick Count(mSec)"=w1403:u32)
      n233 = Equal?(x=w1398, y=w1397) -> (x = y?=w1396:bool)
      n234 = Not Equal?(x=w1397, y=w1390) -> (x != y?=w1395:bool)
      n235 = case shown="False" w1404 {
        selector: w1404 -> [w1415 w1453]
        tunnel: w1409 -> [w1422 w1460]
        tunnel: w1408 -> [w1420 w1458]
        tunnel: w1407 -> [w1418 w1456]
        tunnel: [w1417 w1455] -> w1406
        tunnel: [w1416 w1454] -> w1405
        tunnel: w1403 -> [w1414 w1452]
        tunnel: [w1413 w1451] -> w1402
        tunnel: [w1412 w1450] -> w1401
        tunnel: w1400 -> [w1411 w1449]
        tunnel: w1399 -> [w1410 _]
        frame False {
          # "Pump is in an off state.  Check\nif it started."
          n236 = Greater?(x=w1422, y="On Current Thresh") -> (0:w1419:bool)
          n237 = case shown="True" w1419 {
            tunnel: w1420 -> [_ w1429]
            tunnel: w1418 -> [w1424 w1435]
            tunnel: [w1424 w1434] -> w1417
            tunnel: w1415 -> [w1426 w1433]
            tunnel: [w1426 w1432] -> w1416
            tunnel: w1414 -> [w1425 w1430]
            tunnel: [w1425 w1431] -> w1413
            tunnel: [w1423 w1428] -> w1412
            tunnel: w1411 -> [w1423 _]
            tunnel: w1410 -> [_ w1427]
            frame False {
              # "Pump is off."
            }
            frame True {
              # "Pump is on, or trying to start."
              n238 = Subtract(x=w1430, y=w1429) -> (x-y=w1428:u32)
              n239 = Greater?(x=w1428, y="Min On Time") -> (0:w1436:bool)
              n240 = case shown="True" w1436 {
                tunnel: w1435 -> [w1440 w1445]
                tunnel: [w1440 w1444] -> w1434
                tunnel: w1433 -> [w1438 _]
                tunnel: [w1438 TRUE] -> w1432
                tunnel: [w1439 w1442] -> w1431
                tunnel: w1430 -> [_ w1442]
                tunnel: w1429 -> [w1439 _]
                tunnel: w1427 -> [_ w1441]
                frame False {
                  # "Pump has NOT met the minimum on time yet."
                }
                frame True {
                  # "Pump has met the minimum on time, so it has started.\nCount this as a successful start."
                  n241 = case shown="True" w1441 {
                    tunnel: w1445 -> [w1446 w1448]
                    tunnel: [w1446 w1447] -> w1444
                    frame False {
                    }
                    frame True {
                      n242 = Increment(x=w1448) -> (x+1=w1447:u32)
                    }
                  }
                }
              }
            }
          }
        }
        frame True {
          # "Pump is in an on state.  Check\nif it stopped."
          n243 = Less?(x=w1460, y="Off Current Thresh") -> (x < y?=w1457:bool)
          n244 = case shown="True" w1457 {
            tunnel: w1458 -> [_ w1466]
            tunnel: w1456 -> [w1463 w1472]
            tunnel: [w1463 w1471] -> w1455
            tunnel: w1453 -> [w1462 w1470]
            tunnel: [w1462 w1469] -> w1454
            tunnel: w1452 -> [w1464 w1467]
            tunnel: [w1464 w1468] -> w1451
            tunnel: [w1461 w1465] -> w1450
            tunnel: w1449 -> [w1461 _]
            frame False {
              # "Pump is in on."
            }
            frame True {
              # "Pump is off, but make sure it's\nacutally off, and not just noise.\nSo, check that current is low\nfor a minimum amount of time."
              n245 = Subtract(x=w1467, y=w1466) -> (x-y=w1465:u32)
              n246 = Greater?(x=w1465, y="Min Off Time") -> (0:w1473:bool)
              n247 = case shown="True" w1473 {
                tunnel: w1472 -> [w1476 w1479]
                tunnel: [w1476 w1479] -> w1471
                tunnel: w1470 -> [w1477 _]
                tunnel: [w1477 FALSE] -> w1469
                tunnel: [w1475 w1478] -> w1468
                tunnel: w1467 -> [_ w1478]
                tunnel: w1466 -> [w1475 _]
                frame False {
                  # "Pump has NOT met the minimum off time yet."
                }
                frame True {
                  # "Pump has met the minimum off time, so it is indeed off."
                }
              }
            }
          }
        }
      }
      n248 = Compound Arithmetic op=AND(w1389, w1396, w1395) -> (w1394:bool)
      n249 = Increment(x=w1392) -> (x+1=w1393:u32)
      n250 = Select(t=w1393, s=w1394, f=w1392) -> (s? t:f=w1391:u32)
    }
    "Actual Pump Starts" <- w1366
    "Timers (ms)" <- w1379
    "Pump On States" <- w1381
    "Cmd Pump Starts" <- w1364
    n251 = To Long Integer(number=w1366) -> (32bit integer=w1365:i32[])
    n252 = To Long Integer(number=w1364) -> (32bit integer=w1363:i32[])
    n253 = Subtract(x=w1365, y=w1363) -> (x-y=→"Restarts":i32[])
  }
  n254 = timed-loop "AI Resample Loop" {
    timing: w48 -> [_]
    timing-out: [_] -> w47
    shift-right: [w1502] -> _
    shift-left: u32 0 ("Sample Divisor") -> [w1489]
    shift-right: [w1501] -> _
    shift-left: w44 -> [w1490]
    tunnel: w45 -> [w1495]
    tunnel: w44 -> [w1494]
    stop <- FALSE stop-if-true
    # "Press, Flow"
    # "Ctrlr Current"
    # "30 items"
    n255 = global read "ADC AI Global.vi" "AI16-47"() -> (w1485:fxp<+/-,28,17>[])
    n256 = global read "Diagnostic Global.vi" "Diag_Global"() -> (w1482:fxp<+/-,28,17>[])
    n257 = local read "Duty (Ticks)"() -> (w1481:i32[])
    n258 = Array Subset(array=w1485, length=6) -> (w1484:fxp<+/-,28,17>[])  [unwired: 1 in]
    n259 = Array Subset(array=w1485, index=14, length=12) -> (w1483:fxp<+/-,28,17>[])
    n260 = Less Or Equal?(x="AI Divisor", y=w1489) -> (x <= y?=w1493:bool)
    n261 = Build Array (concatenate)(w1484, w1483, w1482, w1481) -> (w1491:fxp<+/-,43,32>[])
    n262 = feedback #16() -> (w1497:fxp<+/-,43,32>[])  [unwired: 1 in]
    n263 = Select(t=w1491, s=w1493, f=w1497) -> (s? t:f=w1496:fxp<+/-,43,32>[])
    n264 = feedback-in #16(w1496) -> ()
    n265 = Less Or Equal?(x=w1490, y=w1495) -> (x <= y?=w1499:bool)
    n266 = Or(x=w1493, y=w1499) -> (x .or. y?=w1492:bool)
    n267 = case shown="True" w1492 {
      tunnel: w1490 -> [_ w1511]
      tunnel: [w1509 w1512] -> w1498
      tunnel: w1496 -> [_ w1510]
      tunnel: w1494 -> [w1509 _]
      frame False {
      }
      frame True {
        n268 = Decrement(x=w1511) -> (x-1=w1512:u8)
        n269 = case shown="1..30" w1512 {
          selector: w1512 -> [w1519 _ _]
          tunnel: [w1517 fxp<+/-,28,17> -9999.0 ("AI0") fxp<+/-,28,17> -5000.0 ("AI0")] -> w1514
          tunnel: [TRUE TRUE FALSE] -> w1513
          tunnel: w1510 -> [w1521 _ _]
          frame 1..30 {
            # "Data case for\nAI Data"
            n270 = Subtract(x=u8 30 ("Sample Divisor"), y=w1519) -> (x-y=w1518:u8)
            n271 = Index Array(array=w1521, index=w1518) -> (element=w1517:fxp<+/-,43,32>)
          }
          frame 0 {
            # "Used to write AI Data\nIndexer"
          }
          frame Default {
            # "Sould never get to\nthis case."
          }
        }
        n272 = case shown="True" w1513 {
          tunnel: w1514 -> [_ w1516]
          frame False {
          }
          frame True {
            n273 = xnode ("FIFO Method Node")("Element"=w1516, "Timeout"=u8 0) -> ()  [unwired: 1 in, 2 out]
          }
        }
      }
    }
    n274 = case shown="False" w1493 {
      tunnel: w1489 -> [w1506 _]
      tunnel: [w1505 u32 0] -> w1502
      tunnel: w1498 -> [w1504 w1507]
      tunnel: [w1504 w1507] -> w1501
      frame False {
        n275 = Increment(x=w1506) -> (x+1=w1505:u32)
      }
      frame True {
      }
    }
  }
  n276 = timed-loop {
    timing: w9 -> [_]
    timing-out: [_] -> w8
    stop <- FALSE stop-if-true
    w1535 = fxp<+/-,28,17>[] [0.0, 0.0, 0.0, 0.0, 0.0, 0.0]  # Speed Placeholder
    n277 = global read "Pump Currents Global.vi" "Pump Currents"() -> (w1533:fxp<+/-,28,17>[])
    n278 = global read "ADC AI Global (Avg).vi" "AI22-47 (Avg)"() -> (w1532:fxp<+/-,28,17>[])
    n279 = local read "Elapsed Times"() -> (→"Elapsed Times OUT":fxp<+,40,40>[])
    n280 = global read "Onboard AIs Global.vi" "Onboard AI's"() -> (w1531:fxp<+/-,28,17>[])
    n281 = global read "Diagnostic Global.vi" "Diag_Global"() -> (w1534:fxp<+/-,28,17>[])
    n282 = Build Array (concatenate)(w1531, w1533, w1535, w1532, w1534) -> (→"Data OUT":fxp<+/-,28,17>[])
  }
  n283 = node-c288(w28) -> ()
  n284 = while {
    stop <- FALSE stop-if-true
    n285 = xnode "FPGA I/O Node"("AO0"="PS Cmd", "AO1"="Pressure Cmd", "AO2"="AO2", "AO3"="AO3") -> ()  [unwired: 5 in, 5 out]
  }
  n286 = while {
    stop <- FALSE stop-if-true
    w1551 = fxp<+/-,28,17> 0.0 ("Controller_Current_1 (AI6)")
    # "set at 100 Hz"
    # "S 28 17"
    # "S 24 5"
    n287 = xnode "FPGA I/O Node"() -> ("Voltage_1 (AI0/8)"=w1557:fxp<+/-,24,5>, "Voltage_2 (AI1/9)"=w1553:fxp<+/-,24,5>, "Voltage_3 (AI2/10)"=w1554:fxp<+/-,24,5>, "Voltage_4 (AI3/11)"=w1552:fxp<+/-,24,5>, "Voltage_5 (AI4/12)"=w1555:fxp<+/-,24,5>, "Voltage_6 (AI5/13)"=w1556:fxp<+/-,24,5>, "Spare_1"=w1564:fxp<+/-,24,5>, "Spare_2"=w1565:fxp<+/-,24,5>, "Spare_3"=w1566:fxp<+/-,24,5>, "PS_Sense (AI15)"=w1567:fxp<+/-,24,5>)  [unwired: 10 in, 10 out]
    n288 = To Fixed-Point(fixed-point type=w1551, number=w1557) -> (fixed-point=w1550:fxp<+/-,28,17>)
    n289 = To Fixed-Point(fixed-point type=w1551, number=w1553) -> (fixed-point=w1549:fxp<+/-,28,17>)
    n290 = To Fixed-Point(fixed-point type=w1551, number=w1554) -> (fixed-point=w1548:fxp<+/-,28,17>)
    n291 = To Fixed-Point(fixed-point type=w1551, number=w1552) -> (fixed-point=w1546:fxp<+/-,28,17>)
    n292 = To Fixed-Point(fixed-point type=w1551, number=w1555) -> (fixed-point=w1545:fxp<+/-,28,17>)
    n293 = To Fixed-Point(fixed-point type=w1551, number=w1556) -> (fixed-point=w1544:fxp<+/-,28,17>)
    n294 = To Fixed-Point(fixed-point type=w1551, number=w1564) -> (fixed-point=w1559:fxp<+/-,28,17>)
    n295 = To Fixed-Point(fixed-point type=w1551, number=w1565) -> (fixed-point=w1560:fxp<+/-,28,17>)
    n296 = To Fixed-Point(fixed-point type=w1551, number=w1566) -> (fixed-point=w1561:fxp<+/-,28,17>)
    n297 = To Fixed-Point(fixed-point type=w1551, number=w1567) -> (fixed-point=w1562:fxp<+/-,28,17>)
    n298 = Build Array(w1550, w1549, w1548, w1546, w1545, w1544, w1559, w1560, w1561, w1562) -> (w1547:fxp<+/-,28,17>[])
    n299 = global write "Onboard AIs Global.vi" "Onboard AI's"(w1547) -> ()
    n300 = call "Wait"("Count(mSec)"=u32 10) -> ()  [unwired: 1 out]
  }
  n301 = node-c288(w8) -> ()
  n302 = while {
    shift-right: [w1578] -> _
    shift-left: 0 ("Moving Point Index") -> [w1579]
    stop <- FALSE stop-if-true
    w1577 = 127 ("N (# of Ave Pts 8 max)")
    # "Ctrl Current, Temp,\nPressure, Flow\nAI22-47"
    # "S 28 17"
    # "set at 1 kHz"
    n303 = global read "Flow Frequencies Global.vi" "Flow Frequencies"() -> (w1568:fxp<+/-,28,17>[])
    n304 = global read "ADC AI Global.vi" "AI16-47"() -> (w1573:fxp<+/-,28,17>[])
    n305 = Array Subset(array=w1573, index=6, length=26) -> (w1570:fxp<+/-,28,17>[])
    n306 = case shown="True" "Freq Flow?" {
      tunnel: w1570 -> [w1585 w1589]
      tunnel: w1568 -> [_ w1588]
      tunnel: [w1585 w1586] -> w1569
      frame False {
      }
      frame True {
        n307 = Replace Array Subset(array=w1589, new element=w1588, index=14) -> (w1586:fxp<+/-,28,17>[])
      }
    }
    n308 = for {
      tunnel: w1579 -> [w1590]
      tunnel: w1577 -> [w1591]
      tunnel: [w1595] -> w1572 mode=indexing
      tunnel: w1569 -> [w1594] mode=indexing
      tunnel: refnum<k21> "Running Avg Memory" ("Memory") -> [w1593]
      i -> [w1592]
      n309 = call "Moving Average.vi"("Memory In"=w1593, "N (# of Ave Pts 127 max)"=w1591, "Moving Point Index"=w1590, "Data IN"=w1594, "Channel#"=w1592) -> ("Averaged Data"=w1595:fxp<+/-,28,17>)  [unwired: 10 in]
    }
    n310 = global write "ADC AI Global (Avg).vi" "AI22-47 (Avg)"(w1572) -> ()
    n311 = Increment(x=w1579) -> (x+1=w1581:i32)
    n312 = Greater Or Equal?(x=w1579, y=w1577) -> (x >= y?=w1580:bool)
    n313 = Select(t=0, s=w1580, f=w1581) -> (s? t:f=w1578:i32)
    n314 = call "Wait2"("Count(mSec)"=u32 1) -> ()  [unwired: 1 out]
  }
  n315 = node-c288(w26) -> ()
  n316 = node-c288() -> (w11:T4)  [unwired: 1 in]
  n317 = timed-loop {
    shift-right: [w1675] -> _
    shift-left: _ -> [w1674]
    shift-right: [w1673] -> _
    shift-left: _ -> [w1672]
    shift-right: [w1670] -> _
    shift-left: _ -> [w1671]
    shift-right: [w1668] -> _
    shift-left: _ -> [w1669]
    timing: w11 -> [_]
    timing-out: [_] -> w10
    shift-right: [w1666] -> _
    shift-left: _ -> [w1667]
    shift-right: [w1657] -> _
    shift-left: _ -> [w1658]
    shift-right: [w1659] -> _
    shift-left: _ -> [w1660]
    shift-right: [w1662] -> _
    shift-left: _ -> [w1661]
    shift-right: [w1664] -> _
    shift-left: _ -> [w1663]
    shift-right: [w1620] -> _
    shift-left: _ -> [w1665]
    shift-right: [w1656] -> _
    shift-left: _ -> [w1655]
    shift-right: [w1654] -> _
    shift-left: _ -> [w1653]
    shift-right: [w1651] -> _
    shift-left: _ -> [w1652]
    shift-right: [w1649] -> _
    shift-left: _ -> [w1650]
    shift-right: [w1619] -> _
    shift-left: _ -> [w1648]
    shift-right: [w1639] -> _
    shift-left: _ -> [w1640]
    shift-right: [w1641] -> _
    shift-left: _ -> [w1642]
    shift-right: [w1644] -> _
    shift-left: _ -> [w1643]
    shift-right: [w1646] -> _
    shift-left: _ -> [w1645]
    shift-right: [w1618] -> _
    shift-left: _ -> [w1647]
    shift-right: [w1638] -> _
    shift-left: _ -> [w1637]
    shift-right: [w1636] -> _
    shift-left: _ -> [w1635]
    shift-right: [w1633] -> _
    shift-left: _ -> [w1634]
    shift-right: [w1631] -> _
    shift-left: _ -> [w1632]
    shift-right: [w1617] -> _
    shift-left: _ -> [w1630]
    shift-right: [w1621] -> _
    shift-left: _ -> [w1622]
    shift-right: [w1623] -> _
    shift-left: _ -> [w1624]
    shift-right: [w1626] -> _
    shift-left: _ -> [w1625]
    shift-right: [w1628] -> _
    shift-left: _ -> [w1627]
    shift-right: [w1616] -> _
    shift-left: _ -> [w1629]
    stop <- FALSE stop-if-true
    n318 = xnode "FPGA I/O Node"() -> ("RMC/DIO38"=w1596:bool)  [unwired: 1 in, 1 out]
    n319 = xnode "FPGA I/O Node"() -> ("RMC/DIO39"=w1614:bool)  [unwired: 1 in, 1 out]
    n320 = xnode "FPGA I/O Node"() -> ("RMC/DIO40"=w1612:bool)  [unwired: 1 in, 1 out]
    n321 = xnode "FPGA I/O Node"() -> ("RMC/DIO41"=w1610:bool)  [unwired: 1 in, 1 out]
    n322 = xnode "FPGA I/O Node"() -> ("RMC/DIO42"=w1608:bool)  [unwired: 1 in, 1 out]
    n323 = xnode "FPGA I/O Node"() -> ("RMC/DIO43"=w1606:bool)  [unwired: 1 in, 1 out]
    n324 = call "FPGA Debounce Digital.vi"("Input Signal"=w1596, "Cycles to Filter"="Diagnostic Filter") -> ("Output Filtered Signal"=w1615:bool)
    n325 = call "FPGA Debounce Digital.vi"("Input Signal"=w1614, "Cycles to Filter"="Diagnostic Filter") -> ("Output Filtered Signal"=w1613:bool)
    n326 = call "FPGA Debounce Digital.vi"("Input Signal"=w1612, "Cycles to Filter"="Diagnostic Filter") -> ("Output Filtered Signal"=w1611:bool)
    n327 = call "FPGA Debounce Digital.vi"("Input Signal"=w1610, "Cycles to Filter"="Diagnostic Filter") -> ("Output Filtered Signal"=w1609:bool)
    n328 = call "FPGA Debounce Digital.vi"("Input Signal"=w1608, "Cycles to Filter"="Diagnostic Filter") -> ("Output Filtered Signal"=w1607:bool)
    n329 = call "FPGA Debounce Digital.vi"("Input Signal"=w1606, "Cycles to Filter"="Diagnostic Filter") -> ("Output Filtered Signal"=w1605:bool)
    n330 = To Fixed-Point(fixed-point type=fxp<+/-,32,32> 0.0 ("s? t:f"), number="Diagnostic Freq Coeff") -> (fixed-point=w1602:fxp<+/-,32,32>)
    n331 = case shown="\"PSA\"" "Diagnostic Mode" {
      tunnel: [w1679 w1822 w2149] -> w1675
      tunnel: w1674 -> [_ w1821 w2150]
      tunnel: [w1677 w1820 w2045] -> w1673
      tunnel: w1672 -> [_ w1819 _]
      tunnel: w1671 -> [_ w1818 _]
      tunnel: [w1679 w1812 w2046] -> w1670
      tunnel: w1669 -> [_ w1811 _]
      tunnel: [w1679 w1810 w2046] -> w1668
      tunnel: w1667 -> [_ w1806 w2151]
      tunnel: [w1678 w1805 w2044] -> w1666
      tunnel: w1665 -> [_ w1804 w2066]
      tunnel: [w1679 w1800 w2046] -> w1664
      tunnel: w1663 -> [_ w1799 _]
      tunnel: [w1679 w1798 w2046] -> w1662
      tunnel: w1661 -> [_ w1792 _]
      tunnel: w1660 -> [_ w1791 _]
      tunnel: [w1677 w1790 w2045] -> w1659
      tunnel: w1658 -> [_ w1789 w2067]
      tunnel: [w1679 w1788 w2065] -> w1657
      tunnel: [w1679 w1777 w2061] -> w1656
      tunnel: w1655 -> [_ w1776 w2063]
      tunnel: [w1677 w1775 w2045] -> w1654
      tunnel: w1653 -> [_ w1774 _]
      tunnel: w1652 -> [_ w1773 _]
      tunnel: [w1679 w1767 w2046] -> w1651
      tunnel: w1650 -> [_ w1766 _]
      tunnel: [w1679 w1765 w2046] -> w1649
      tunnel: w1648 -> [_ w1761 w2062]
      tunnel: w1647 -> [_ w1760 w2059]
      tunnel: [w1679 w1756 w2046] -> w1646
      tunnel: w1645 -> [_ w1755 _]
      tunnel: [w1679 w1754 w2046] -> w1644
      tunnel: w1643 -> [_ w1748 _]
      tunnel: w1642 -> [_ w1747 _]
      tunnel: [w1677 w1746 w2045] -> w1641
      tunnel: w1640 -> [_ w1745 w2057]
      tunnel: [w1679 w1744 w2058] -> w1639
      tunnel: [w1679 w1733 w2053] -> w1638
      tunnel: w1637 -> [_ w1732 w2055]
      tunnel: [w1677 w1731 w2045] -> w1636
      tunnel: w1635 -> [_ w1730 _]
      tunnel: w1634 -> [_ w1729 _]
      tunnel: [w1679 w1723 w2046] -> w1633
      tunnel: w1632 -> [_ w1722 _]
      tunnel: [w1679 w1721 w2046] -> w1631
      tunnel: w1630 -> [_ w1717 w2054]
      tunnel: w1629 -> [_ w1716 w2048]
      tunnel: [w1679 w1712 w2046] -> w1628
      tunnel: w1627 -> [_ w1711 _]
      tunnel: [w1679 w1710 w2046] -> w1626
      tunnel: w1625 -> [_ w1704 _]
      tunnel: w1624 -> [_ w1703 _]
      tunnel: [w1677 w1702 w2045] -> w1623
      tunnel: w1622 -> [_ w1701 w2049]
      tunnel: [w1679 w1700 w2047] -> w1621
      tunnel: [w1678 w1694 w2043] -> w1620
      tunnel: [w1678 w1693 w2042] -> w1619
      tunnel: [w1678 w1692 w2041] -> w1618
      tunnel: [w1678 w1691 w2040] -> w1617
      tunnel: [w1678 w1690 w2039] -> w1616
      tunnel: w1615 -> [_ w1689 w2152]
      tunnel: w1613 -> [_ w1688 w2068]
      tunnel: w1611 -> [_ w1687 w2064]
      tunnel: w1609 -> [_ w1686 w2060]
      tunnel: w1607 -> [_ w1685 w2056]
      tunnel: w1605 -> [_ w1684 w2050]
      tunnel: w1602 -> [_ w1683 _]
      tunnel: "Invert Diagnostic" -> [_ w1682 _]
      tunnel: "Diag Max Period (ticks)" -> [_ _ w2051]
      tunnel: [fxp<+/-,28,17>[] [0.0, 0.0, 0.0, 0.0, 0.0, 0.0] w1681 w2038] -> w1597
      frame "None", Default {
        w1677 = FALSE ("Output Filtered Signal")
        w1678 = fxp<+/-,28,17> 0.0 ("AI0")
        w1679 = u32 0 ("f")
      }
      frame "PSA" {
        # "PWM diagnostic code."
        n332 = call "Tick Count2"() -> ("Tick Count(Ticks)"=w1827:u32)
        n333 = call "Tick Count3"() -> ("Tick Count(Ticks)"=w1783:u32)
        n334 = call "Tick Count4"() -> ("Tick Count(Ticks)"=w1782:u32)
        n335 = call "Tick Count5"() -> ("Tick Count(Ticks)"=w1739:u32)
        n336 = call "Tick Count6"() -> ("Tick Count(Ticks)"=w1738:u32)
        n337 = call "Tick Count7"() -> ("Tick Count(Ticks)"=w1695:u32)
        n338 = Greater?(x=w1689, y=w1819) -> (0:w1824:bool)
        n339 = Greater?(x=w1688, y=w1791) -> (0:w1786:bool)
        n340 = Greater?(x=w1687, y=w1774) -> (0:w1779:bool)
        n341 = Greater?(x=w1686, y=w1747) -> (0:w1742:bool)
        n342 = Greater?(x=w1685, y=w1730) -> (0:w1735:bool)
        n343 = Greater?(x=w1684, y=w1703) -> (0:w1698:bool)
        n344 = Subtract(x=w1827, y=w1821) -> (x-y=w1826:u32)
        n345 = Subtract(x=w1783, y=w1789) -> (x-y=w1784:u32)
        n346 = Subtract(x=w1782, y=w1776) -> (x-y=w1781:u32)
        n347 = Subtract(x=w1739, y=w1745) -> (x-y=w1740:u32)
        n348 = Subtract(x=w1738, y=w1732) -> (x-y=w1737:u32)
        n349 = Subtract(x=w1695, y=w1701) -> (x-y=w1696:u32)
        n350 = Less?(x=w1689, y=w1819) -> (x < y?=w1825:bool)
        n351 = Less?(x=w1688, y=w1791) -> (x < y?=w1785:bool)
        n352 = Less?(x=w1687, y=w1774) -> (x < y?=w1780:bool)
        n353 = Less?(x=w1686, y=w1747) -> (x < y?=w1741:bool)
        n354 = Less?(x=w1685, y=w1730) -> (x < y?=w1736:bool)
        n355 = Less?(x=w1684, y=w1703) -> (x < y?=w1697:bool)
        n356 = case shown="True" w1682 {
          tunnel: w1825 -> [w2034 w2036]
          tunnel: w1824 -> [w2033 w2037]
          tunnel: [w2034 w2037] -> w1823
          tunnel: [w2033 w2036] -> w1809
          tunnel: w1689 -> [w2032 w2035]
          tunnel: [w2032 w2035] -> w1820
          frame False {
          }
          frame True {
          }
        }
        n357 = case shown="True" w1682 {
          tunnel: w1785 -> [w1999 w2001]
          tunnel: w1786 -> [w1998 w2002]
          tunnel: [w1999 w2002] -> w1787
          tunnel: [w1998 w2001] -> w1801
          tunnel: w1688 -> [w1997 w2000]
          tunnel: [w1997 w2000] -> w1790
          frame False {
          }
          frame True {
          }
        }
        n358 = case shown="True" w1682 {
          tunnel: w1780 -> [w1964 w1966]
          tunnel: w1779 -> [w1963 w1967]
          tunnel: [w1964 w1967] -> w1778
          tunnel: [w1963 w1966] -> w1764
          tunnel: w1687 -> [w1962 w1965]
          tunnel: [w1962 w1965] -> w1775
          frame False {
          }
          frame True {
          }
        }
        n359 = case shown="True" w1682 {
          tunnel: w1741 -> [w1929 w1931]
          tunnel: w1742 -> [w1928 w1932]
          tunnel: [w1929 w1932] -> w1743
          tunnel: [w1928 w1931] -> w1757
          tunnel: w1686 -> [w1927 w1930]
          tunnel: [w1927 w1930] -> w1746
          frame False {
          }
          frame True {
          }
        }
        n360 = case shown="True" w1682 {
          tunnel: w1736 -> [w1894 w1896]
          tunnel: w1735 -> [w1893 w1897]
          tunnel: [w1894 w1897] -> w1734
          tunnel: [w1893 w1896] -> w1720
          tunnel: w1685 -> [w1892 w1895]
          tunnel: [w1892 w1895] -> w1731
          frame False {
          }
          frame True {
          }
        }
        n361 = case shown="True" w1682 {
          tunnel: w1697 -> [w1859 w1861]
          tunnel: w1698 -> [w1858 w1862]
          tunnel: [w1859 w1862] -> w1699
          tunnel: [w1858 w1861] -> w1713
          tunnel: w1684 -> [w1857 w1860]
          tunnel: [w1857 w1860] -> w1702
          frame False {
          }
          frame True {
          }
        }
        n362 = Select(t=w1826, s=w1823, f=w1818) -> (s? t:f=w1812:u32)
        n363 = Select(t=w1784, s=w1787, f=w1792) -> (s? t:f=w1798:u32)
        n364 = Select(t=w1781, s=w1778, f=w1773) -> (s? t:f=w1767:u32)
        n365 = Select(t=w1740, s=w1743, f=w1748) -> (s? t:f=w1754:u32)
        n366 = Select(t=w1737, s=w1734, f=w1729) -> (s? t:f=w1723:u32)
        n367 = Select(t=w1696, s=w1699, f=w1704) -> (s? t:f=w1710:u32)
        n368 = Select(t=w1827, s=w1809, f=w1821) -> (s? t:f=w1822:u32)
        n369 = Select(t=w1783, s=w1801, f=w1789) -> (s? t:f=w1788:u32)
        n370 = Select(t=w1782, s=w1764, f=w1776) -> (s? t:f=w1777:u32)
        n371 = Select(t=w1739, s=w1757, f=w1745) -> (s? t:f=w1744:u32)
        n372 = Select(t=w1738, s=w1720, f=w1732) -> (s? t:f=w1733:u32)
        n373 = Select(t=w1695, s=w1713, f=w1701) -> (s? t:f=w1700:u32)
        n374 = Select(t=w1812, s=w1809, f=w1811) -> (s? t:f=w1810:u32)
        n375 = Select(t=w1798, s=w1801, f=w1799) -> (s? t:f=w1800:u32)
        n376 = Select(t=w1767, s=w1764, f=w1766) -> (s? t:f=w1765:u32)
        n377 = Select(t=w1754, s=w1757, f=w1755) -> (s? t:f=w1756:u32)
        n378 = Select(t=w1723, s=w1720, f=w1722) -> (s? t:f=w1721:u32)
        n379 = Select(t=w1710, s=w1713, f=w1711) -> (s? t:f=w1712:u32)
        n380 = To Fixed-Point(fixed-point type=fxp<+/-,32,32> 0.0 ("s? t:f"), number=w1810) -> (fixed-point=w1813:fxp<+/-,32,32>)
        n381 = To Fixed-Point(fixed-point type=fxp<+/-,32,32> 0.0 ("s? t:f"), number=w1800) -> (fixed-point=w1797:fxp<+/-,32,32>)
        n382 = To Fixed-Point(fixed-point type=fxp<+/-,32,32> 0.0 ("s? t:f"), number=w1765) -> (fixed-point=w1768:fxp<+/-,32,32>)
        n383 = To Fixed-Point(fixed-point type=fxp<+/-,32,32> 0.0 ("s? t:f"), number=w1756) -> (fixed-point=w1753:fxp<+/-,32,32>)
        n384 = To Fixed-Point(fixed-point type=fxp<+/-,32,32> 0.0 ("s? t:f"), number=w1721) -> (fixed-point=w1724:fxp<+/-,32,32>)
        n385 = To Fixed-Point(fixed-point type=fxp<+/-,32,32> 0.0 ("s? t:f"), number=w1712) -> (fixed-point=w1709:fxp<+/-,32,32>)
        n386 = feedback #17() -> (w1814:bool)  [unwired: 1 in]
        n387 = And(x=w1809, y=w1814) -> (x .and. y?=w1815:bool)
        n388 = feedback #18() -> (w1796:bool)  [unwired: 1 in]
        n389 = And(x=w1801, y=w1796) -> (x .and. y?=w1795:bool)
        n390 = feedback #19() -> (w1769:bool)  [unwired: 1 in]
        n391 = And(x=w1764, y=w1769) -> (x .and. y?=w1770:bool)
        n392 = feedback #20() -> (w1752:bool)  [unwired: 1 in]
        n393 = And(x=w1757, y=w1752) -> (x .and. y?=w1751:bool)
        n394 = feedback #21() -> (w1725:bool)  [unwired: 1 in]
        n395 = And(x=w1720, y=w1725) -> (x .and. y?=w1726:bool)
        n396 = feedback #22() -> (w1708:bool)  [unwired: 1 in]
        n397 = And(x=w1713, y=w1708) -> (x .and. y?=w1707:bool)
        n398 = xnode "High Throughput Divide"("x"=w1813, "y"=w1683, "input valid"=w1815) -> ("x/y"=w1808:fxp<+/-,28,17>, "output valid"=w1807:bool, "ready for input"=w1816:bool)  [unwired: 1 in]
        n399 = feedback-in #17(w1816) -> ()
        n400 = xnode "High Throughput Divide"("x"=w1797, "y"=w1683, "input valid"=w1795) -> ("x/y"=w1802:fxp<+/-,28,17>, "output valid"=w1803:bool, "ready for input"=w1794:bool)  [unwired: 1 in]
        n401 = feedback-in #18(w1794) -> ()
        n402 = xnode "High Throughput Divide"("x"=w1768, "y"=w1683, "input valid"=w1770) -> ("x/y"=w1763:fxp<+/-,28,17>, "output valid"=w1762:bool, "ready for input"=w1771:bool)  [unwired: 1 in]
        n403 = feedback-in #19(w1771) -> ()
        n404 = xnode "High Throughput Divide"("x"=w1753, "y"=w1683, "input valid"=w1751) -> ("x/y"=w1758:fxp<+/-,28,17>, "output valid"=w1759:bool, "ready for input"=w1750:bool)  [unwired: 1 in]
        n405 = feedback-in #20(w1750) -> ()
        n406 = xnode "High Throughput Divide"("x"=w1724, "y"=w1683, "input valid"=w1726) -> ("x/y"=w1719:fxp<+/-,28,17>, "output valid"=w1718:bool, "ready for input"=w1727:bool)  [unwired: 1 in]
        n407 = feedback-in #21(w1727) -> ()
        n408 = xnode "High Throughput Divide"("x"=w1709, "y"=w1683, "input valid"=w1707) -> ("x/y"=w1714:fxp<+/-,28,17>, "output valid"=w1715:bool, "ready for input"=w1706:bool)  [unwired: 1 in]
        n409 = feedback-in #22(w1706) -> ()
        n410 = Select(t=w1808, s=w1807, f=w1806) -> (s? t:f=w1805:fxp<+/-,28,17>)
        n411 = Select(t=w1802, s=w1803, f=w1804) -> (s? t:f=w1694:fxp<+/-,28,17>)
        n412 = Select(t=w1763, s=w1762, f=w1761) -> (s? t:f=w1693:fxp<+/-,28,17>)
        n413 = Select(t=w1758, s=w1759, f=w1760) -> (s? t:f=w1692:fxp<+/-,28,17>)
        n414 = Select(t=w1719, s=w1718, f=w1717) -> (s? t:f=w1691:fxp<+/-,28,17>)
        n415 = Select(t=w1714, s=w1715, f=w1716) -> (s? t:f=w1690:fxp<+/-,28,17>)
        n416 = Build Array(w1805, w1694, w1693, w1692, w1691, w1690) -> (w1681:fxp<+/-,28,17>[])
      }
      frame "CMFB" {
        w2045 = FALSE ("Output Filtered Signal")
        w2046 = u32 0
        w2052 = fxp<+,32,32> 40000000.0 ("x")
        # "CMFB diagnostic code."
        n417 = feedback #23() -> (w2168:bool)  [unwired: 1 in]
        n418 = feedback-in #23(w2152) -> ()
        n419 = feedback #24() -> (w2133:bool)  [unwired: 1 in]
        n420 = feedback-in #24(w2068) -> ()
        n421 = feedback #25() -> (w2132:bool)  [unwired: 1 in]
        n422 = feedback-in #25(w2064) -> ()
        n423 = feedback #26() -> (w2101:bool)  [unwired: 1 in]
        n424 = feedback-in #26(w2060) -> ()
        n425 = feedback #27() -> (w2100:bool)  [unwired: 1 in]
        n426 = feedback-in #27(w2056) -> ()
        n427 = feedback #28() -> (w2069:bool)  [unwired: 1 in]
        n428 = feedback-in #28(w2050) -> ()
        n429 = Increment(x=w2150) -> (x+1=w2165:u32)
        n430 = Increment(x=w2067) -> (x+1=w2136:u32)
        n431 = Increment(x=w2063) -> (x+1=w2129:u32)
        n432 = Increment(x=w2057) -> (x+1=w2104:u32)
        n433 = Increment(x=w2055) -> (x+1=w2097:u32)
        n434 = Increment(x=w2049) -> (x+1=w2072:u32)
        n435 = Greater?(x=w2152, y=w2168) -> (0:w2153:bool)
        n436 = Greater?(x=w2068, y=w2133) -> (0:w2148:bool)
        n437 = Greater?(x=w2064, y=w2132) -> (0:w2117:bool)
        n438 = Greater?(x=w2060, y=w2101) -> (0:w2116:bool)
        n439 = Greater?(x=w2056, y=w2100) -> (0:w2085:bool)
        n440 = Greater?(x=w2050, y=w2069) -> (0:w2084:bool)
        n441 = Greater?(x=w2165, y=w2051) -> (0:w2167:bool)
        n442 = Greater?(x=w2136, y=w2051) -> (0:w2134:bool)
        n443 = Greater?(x=w2129, y=w2051) -> (0:w2131:bool)
        n444 = Greater?(x=w2104, y=w2051) -> (0:w2102:bool)
        n445 = Greater?(x=w2097, y=w2051) -> (0:w2099:bool)
        n446 = Greater?(x=w2072, y=w2051) -> (0:w2070:bool)
        n447 = To Fixed-Point(number=w2165) -> (fixed-point=w2164:fxp<+,32,32>)  [unwired: 1 in]
        n448 = To Fixed-Point(number=w2136) -> (fixed-point=w2137:fxp<+,32,32>)  [unwired: 1 in]
        n449 = To Fixed-Point(number=w2129) -> (fixed-point=w2128:fxp<+,32,32>)  [unwired: 1 in]
        n450 = To Fixed-Point(number=w2104) -> (fixed-point=w2105:fxp<+,32,32>)  [unwired: 1 in]
        n451 = To Fixed-Point(number=w2097) -> (fixed-point=w2096:fxp<+,32,32>)  [unwired: 1 in]
        n452 = To Fixed-Point(number=w2072) -> (fixed-point=w2073:fxp<+,32,32>)  [unwired: 1 in]
        n453 = feedback #29() -> (w2154:bool)  [unwired: 1 in]
        n454 = And(x=w2153, y=w2154) -> (x .and. y?=w2155:bool)
        n455 = feedback #30() -> (w2147:bool)  [unwired: 1 in]
        n456 = And(x=w2148, y=w2147) -> (x .and. y?=w2146:bool)
        n457 = feedback #31() -> (w2118:bool)  [unwired: 1 in]
        n458 = And(x=w2117, y=w2118) -> (x .and. y?=w2119:bool)
        n459 = feedback #32() -> (w2115:bool)  [unwired: 1 in]
        n460 = And(x=w2116, y=w2115) -> (x .and. y?=w2114:bool)
        n461 = feedback #33() -> (w2086:bool)  [unwired: 1 in]
        n462 = And(x=w2085, y=w2086) -> (x .and. y?=w2087:bool)
        n463 = feedback #34() -> (w2083:bool)  [unwired: 1 in]
        n464 = And(x=w2084, y=w2083) -> (x .and. y?=w2082:bool)
        n465 = xnode "High Throughput Divide"("x"=w2052, "y"=w2164, "input valid"=w2155) -> ("x/y"=w2161:fxp<+,28,17>, "output valid"=w2157:bool, "ready for input"=w2156:bool)  [unwired: 1 in]
        n466 = feedback-in #29(w2156) -> ()
        n467 = xnode "High Throughput Divide"("x"=w2052, "y"=w2137, "input valid"=w2146) -> ("x/y"=w2140:fxp<+,28,17>, "output valid"=w2144:bool, "ready for input"=w2145:bool)  [unwired: 1 in]
        n468 = feedback-in #30(w2145) -> ()
        n469 = xnode "High Throughput Divide"("x"=w2052, "y"=w2128, "input valid"=w2119) -> ("x/y"=w2125:fxp<+,28,17>, "output valid"=w2121:bool, "ready for input"=w2120:bool)  [unwired: 1 in]
        n470 = feedback-in #31(w2120) -> ()
        n471 = xnode "High Throughput Divide"("x"=w2052, "y"=w2105, "input valid"=w2114) -> ("x/y"=w2108:fxp<+,28,17>, "output valid"=w2112:bool, "ready for input"=w2113:bool)  [unwired: 1 in]
        n472 = feedback-in #32(w2113) -> ()
        n473 = xnode "High Throughput Divide"("x"=w2052, "y"=w2096, "input valid"=w2087) -> ("x/y"=w2093:fxp<+,28,17>, "output valid"=w2089:bool, "ready for input"=w2088:bool)  [unwired: 1 in]
        n474 = feedback-in #33(w2088) -> ()
        n475 = xnode "High Throughput Divide"("x"=w2052, "y"=w2073, "input valid"=w2082) -> ("x/y"=w2076:fxp<+,28,17>, "output valid"=w2080:bool, "ready for input"=w2081:bool)  [unwired: 1 in]
        n476 = feedback-in #34(w2081) -> ()
        n477 = Select(t=u32 0 ("f"), s=w2157, f=w2165) -> (s? t:f=w2149:u32)
        n478 = Select(t=u32 0 ("f"), s=w2144, f=w2136) -> (s? t:f=w2065:u32)
        n479 = Select(t=u32 0 ("f"), s=w2121, f=w2129) -> (s? t:f=w2061:u32)
        n480 = Select(t=u32 0 ("f"), s=w2112, f=w2104) -> (s? t:f=w2058:u32)
        n481 = Select(t=u32 0 ("f"), s=w2089, f=w2097) -> (s? t:f=w2053:u32)
        n482 = Select(t=u32 0 ("f"), s=w2080, f=w2072) -> (s? t:f=w2047:u32)
        n483 = To Fixed-Point(fixed-point type=fxp<+/-,28,17> 0.0 ("AI0"), number=w2161) -> (fixed-point=w2159:fxp<+/-,28,17>)
        n484 = To Fixed-Point(fixed-point type=fxp<+/-,28,17> 0.0 ("AI0"), number=w2140) -> (fixed-point=w2142:fxp<+/-,28,17>)
        n485 = To Fixed-Point(fixed-point type=fxp<+/-,28,17> 0.0 ("AI0"), number=w2125) -> (fixed-point=w2123:fxp<+/-,28,17>)
        n486 = To Fixed-Point(fixed-point type=fxp<+/-,28,17> 0.0 ("AI0"), number=w2108) -> (fixed-point=w2110:fxp<+/-,28,17>)
        n487 = To Fixed-Point(fixed-point type=fxp<+/-,28,17> 0.0 ("AI0"), number=w2093) -> (fixed-point=w2091:fxp<+/-,28,17>)
        n488 = To Fixed-Point(fixed-point type=fxp<+/-,28,17> 0.0 ("AI0"), number=w2076) -> (fixed-point=w2078:fxp<+/-,28,17>)
        n489 = Or(x=w2167, y=w2157) -> (x .or. y?=w2162:bool)
        n490 = Or(x=w2134, y=w2144) -> (x .or. y?=w2139:bool)
        n491 = Or(x=w2131, y=w2121) -> (x .or. y?=w2126:bool)
        n492 = Or(x=w2102, y=w2112) -> (x .or. y?=w2107:bool)
        n493 = Or(x=w2099, y=w2089) -> (x .or. y?=w2094:bool)
        n494 = Or(x=w2070, y=w2080) -> (x .or. y?=w2075:bool)
        n495 = Select(t=fxp<+/-,28,17> 0.0 ("AI0"), s=w2167, f=w2159) -> (s? t:f=w2163:fxp<+/-,28,17>)
        n496 = Select(t=fxp<+/-,28,17> 0.0 ("AI0"), s=w2134, f=w2142) -> (s? t:f=w2138:fxp<+/-,28,17>)
        n497 = Select(t=fxp<+/-,28,17> 0.0 ("AI0"), s=w2131, f=w2123) -> (s? t:f=w2127:fxp<+/-,28,17>)
        n498 = Select(t=fxp<+/-,28,17> 0.0 ("AI0"), s=w2102, f=w2110) -> (s? t:f=w2106:fxp<+/-,28,17>)
        n499 = Select(t=fxp<+/-,28,17> 0.0 ("AI0"), s=w2099, f=w2091) -> (s? t:f=w2095:fxp<+/-,28,17>)
        n500 = Select(t=fxp<+/-,28,17> 0.0 ("AI0"), s=w2070, f=w2078) -> (s? t:f=w2074:fxp<+/-,28,17>)
        n501 = Select(t=w2163, s=w2162, f=w2151) -> (s? t:f=w2044:fxp<+/-,28,17>)
        n502 = Select(t=w2138, s=w2139, f=w2066) -> (s? t:f=w2043:fxp<+/-,28,17>)
        n503 = Select(t=w2127, s=w2126, f=w2062) -> (s? t:f=w2042:fxp<+/-,28,17>)
        n504 = Select(t=w2106, s=w2107, f=w2059) -> (s? t:f=w2041:fxp<+/-,28,17>)
        n505 = Select(t=w2095, s=w2094, f=w2054) -> (s? t:f=w2040:fxp<+/-,28,17>)
        n506 = Select(t=w2074, s=w2075, f=w2048) -> (s? t:f=w2039:fxp<+/-,28,17>)
        n507 = Build Array(w2044, w2043, w2042, w2041, w2040, w2039) -> (w2038:fxp<+/-,28,17>[])
      }
    }
    n508 = global write "Diagnostic Global.vi" "Diag_Global"(w1597) -> ()
  }
  n509 = while {
    shift-right: [w2358] -> _
    shift-left: _ -> [w2353]
    stop <- FALSE stop-if-true
    w2345 = refnum<k21> "Signal for Speed"  # FIFO
    # "set at 31.25 kHz"
    n510 = global read "ADC AI Global.vi" "AI16-47"() -> (w2352:fxp<+/-,28,17>[])
    n511 = case shown="1..2500" w2353 {
      tunnel: [fxp<+/-,28,17> -21.0 ("Controller_Current_1 (AI6)") w2398 fxp<+/-,28,17> -22.0 ("Controller_Current_1 (AI6)") w2407 fxp<+/-,28,17> -23.0 ("Controller_Current_1 (AI6)") w2417 fxp<+/-,28,17> -24.0 ("Controller_Current_1 (AI6)") w2426 fxp<+/-,28,17> -25.0 ("Controller_Current_1 (AI6)") w2435 fxp<+/-,28,17> -26.0 ("Controller_Current_1 (AI6)") w2443 fxp<+/-,28,17> -21.5 ("Controller_Current_1 (AI6)") w2452 fxp<+/-,28,17> -22.5 ("Controller_Current_1 (AI6)") w2461 fxp<+/-,28,17> -23.5 ("Controller_Current_1 (AI6)") w2471 fxp<+/-,28,17> -24.5 ("Controller_Current_1 (AI6)") w2480 fxp<+/-,28,17> -25.5 ("Controller_Current_1 (AI6)") w2489 fxp<+/-,28,17> -26.5 ("Controller_Current_1 (AI6)") w2497 fxp<+/-,28,17> -31.0 ("Controller_Current_1 (AI6)")] -> w2349
      tunnel: w2352 -> [_ w2399 _ w2408 _ w2416 _ w2425 _ w2434 _ w2444 _ w2453 _ w2462 _ w2470 _ w2479 _ w2488 _ w2498 _]
      tunnel: [TRUE FALSE TRUE FALSE TRUE FALSE TRUE FALSE TRUE FALSE TRUE FALSE TRUE FALSE TRUE FALSE TRUE FALSE TRUE FALSE TRUE FALSE TRUE FALSE TRUE] -> w2348
      tunnel: "FFT_Amp?" -> [_ w2393 _ w2402 _ w2411 _ w2420 _ w2429 _ w2438 _ w2447 _ w2456 _ w2465 _ w2474 _ w2483 _ w2492 _]
      frame 0, Default {
        # "Start V1"
      }
      frame 1..2500 {
        n512 = Select(t=0 ("index"), s=w2393, f=26) -> (s? t:f=w2395:i32)
        n513 = Index Array(array=w2399, index=w2395) -> (element=w2398:fxp<+/-,28,17>)
      }
      frame 2501 {
        # "Start V2"
      }
      frame 2502..5001 {
        n514 = Select(t=1 ("index"), s=w2402, f=27) -> (s? t:f=w2404:i32)
        n515 = Index Array(array=w2408, index=w2404) -> (element=w2407:fxp<+/-,28,17>)
      }
      frame 5002 {
        # "Start V3"
      }
      frame 5003..7502 {
        n516 = Select(t=2 ("index"), s=w2411, f=28) -> (s? t:f=w2413:i32)
        n517 = Index Array(array=w2416, index=w2413) -> (element=w2417:fxp<+/-,28,17>)
      }
      frame 7503 {
        # "Start V4"
      }
      frame 7504..10003 {
        n518 = Select(t=3 ("index"), s=w2420, f=29) -> (s? t:f=w2422:i32)
        n519 = Index Array(array=w2425, index=w2422) -> (element=w2426:fxp<+/-,28,17>)
      }
      frame 10004 {
        # "Start V5"
      }
      frame 10005..12504 {
        n520 = Select(t=4 ("index"), s=w2429, f=30) -> (s? t:f=w2431:i32)
        n521 = Index Array(array=w2434, index=w2431) -> (element=w2435:fxp<+/-,28,17>)
      }
      frame 12505 {
        # "Start V6"
      }
      frame 12506..15005 {
        n522 = Select(t=5 ("index"), s=w2438, f=31) -> (s? t:f=w2440:i32)
        n523 = Index Array(array=w2444, index=w2440) -> (element=w2443:fxp<+/-,28,17>)
      }
      frame 15006 {
        # "Start V1\nsecond\nread"
      }
      frame 15007..17506 {
        n524 = Select(t=0 ("index"), s=w2447, f=26) -> (s? t:f=w2449:i32)
        n525 = Index Array(array=w2453, index=w2449) -> (element=w2452:fxp<+/-,28,17>)
      }
      frame 17507 {
        # "Start V2\nsecond\nread"
      }
      frame 17508..20007 {
        n526 = Select(t=1 ("index"), s=w2456, f=27) -> (s? t:f=w2458:i32)
        n527 = Index Array(array=w2462, index=w2458) -> (element=w2461:fxp<+/-,28,17>)
      }
      frame 20008 {
        # "Start V3\nSecond\nread"
      }
      frame 20009..22508 {
        n528 = Select(t=2 ("index"), s=w2465, f=28) -> (s? t:f=w2467:i32)
        n529 = Index Array(array=w2470, index=w2467) -> (element=w2471:fxp<+/-,28,17>)
      }
      frame 22509 {
        # "Start V4\nsecond\nread"
      }
      frame 22510..25009 {
        n530 = Select(t=3 ("index"), s=w2474, f=29) -> (s? t:f=w2476:i32)
        n531 = Index Array(array=w2479, index=w2476) -> (element=w2480:fxp<+/-,28,17>)
      }
      frame 25010 {
        # "Start V5\nsecond\nread"
      }
      frame 25011..27510 {
        n532 = Select(t=4 ("index"), s=w2483, f=30) -> (s? t:f=w2485:i32)
        n533 = Index Array(array=w2488, index=w2485) -> (element=w2489:fxp<+/-,28,17>)
      }
      frame 27511 {
        # "Start V6\nsecond\nread"
      }
      frame 27512..30011 {
        n534 = Select(t=5 ("index"), s=w2492, f=31) -> (s? t:f=w2494:i32)
        n535 = Index Array(array=w2498, index=w2494) -> (element=w2497:fxp<+/-,28,17>)
      }
      frame 30012.. {
        # "Hold"
      }
    }
    n536 = xnode "High Throughput Divide"("x"=w2349, "y"=fxp<+,14,14> 13107.0 ("Controller_Current_1 (AI6)")) -> ("x/y"=w2350:fxp<+/-,28,17>)
    n537 = Select(t=w2349, s=w2348, f=w2350) -> (s? t:f=w2347:fxp<+/-,28,17>)
    n538 = To Fixed-Point(fixed-point type=fxp<+/-,25,6> 0.0 ("Controller_Current_1 (AI6)"), number=w2347) -> (fixed-point=w2355:fxp<+/-,25,6>)
    n539 = Increment(x=w2353) -> (x+1=w2359:i32)
    n540 = xnode ("FIFO Write")("Element"=w2355, "Timeout"=0, "FIFO In"=w2345) -> ()  [unwired: 2 out]
    n541 = Greater?(x=w2359, y=31249) -> (0:w2361:bool)
    n542 = call "Wait4"("Count(Ticks)"=u32 1280 ("Count(mSec)")) -> ()  [unwired: 1 out]
    n543 = Select(t=0, s=w2361, f=w2359) -> (s? t:f=w2358:i32)
  }
  n544 = node-c288(w47) -> ()
  n545 = node-c288(w10) -> ()
  n546 = node-c288(w41) -> ()
